vi "PSUSettingsMenu.vi"(8 "error in (no error)":errorcluster, 9 "PSU Calc":T1={"Low speed (km/s)"=2000.0, "High speed (km/s)"=3000.0, "Window (Delta-T)"=0.0, "Lower Cutoff"=0.0, "Multiplier"=0, "Low Charge (fC)"=2000.0, "High Charge (fC)"=2000.0, "High Mass (kg)"=2000.0, "Low Mass (kg)"=2000.0, "High Radius (µm) "=0.0, "Low Radius (µm)"=2000.0, "Exp. Voltage (MV)"=2000.0} {"Exp. Voltage (MV)" step=0.01 format="%#.6f"; "Window (Delta-T)" step=1.0 format="%#.0f"; "High Radius (µm)" min=0.0 max=1000.0; "High Mass (kg)" min=0.0 max=1.0; "High Charge (fC)" min=0.0 max=1000000000000.0; "High speed (km/s)" min=0.0 max=299790.0; "Low speed (km/s)" min=0.0 max=299790.0; "Low Charge (fC)" min=0.0 max=1000000000000.0; "Low Mass (kg)" min=0.0 max=1.0; "Low Radius (µm)" min=0.0 max=299792000.0; "Lower Cutoff" step=1.0 format="%#.0f"; "Multiplier" items=["1k", "10k"]}, 10 "sub vi?":bool, 11 "Enable":bool=TRUE) -> (0 "error out":errorcluster, 1 "OK":bool, 3 "Cancel 2":bool caption="Cancel")   [LabVIEW 2013]
doc: "Displays a standard dialog box that prompts users to enter information, such as a user name and password.\n--------------------\n\nThis Express VI is configured as follows:\n\nMessage to Display to the User:Please Enter Experiment Settings Information For Database Storage.\nThe inputs are: \nNumber: Please Enter Group ID\nText Entry Box: Please Enter Tags:\nText Entry Box: Please Enter Experiment Description:"
uses:
  Controls/PSU Calc.ctl
  <vilib>/Utility/miscctls.llb/LVPointTypeDef.ctl
  <vilib>/addons/database/Connection.llb/Conn Execute.vi
  <vilib>/addons/database/Recordset.llb/Rec Fetch Recordset Data (R).vi
  <vilib>/addons/database/Recordset.llb/Rec Destroy - Connection.vi
  Unused/PSU updated.vi
  <vilib>/addons/database/_DB Variant To Data/Database Variant To Data.xnode
  <vilib>/addons/database/NI_Database_API.lvlib
panel:
  in  "Accept All Particles":bool caption="OK2"
  out "Dust Density\n(g/cc)":dbl
  in  "Variable 2":enum32{"Velocity", "Charge", "Mass"}(radio)
  in  "Variable 1":enum32{"Velocity", "Charge", "Mass"}(radio)
  in  "PSU update":bool caption="OK2"
  in  "Cancel":bool
  in  "OK1":bool
  # "Please Enter PSU Settings For Storage in the CCLDAS Database."
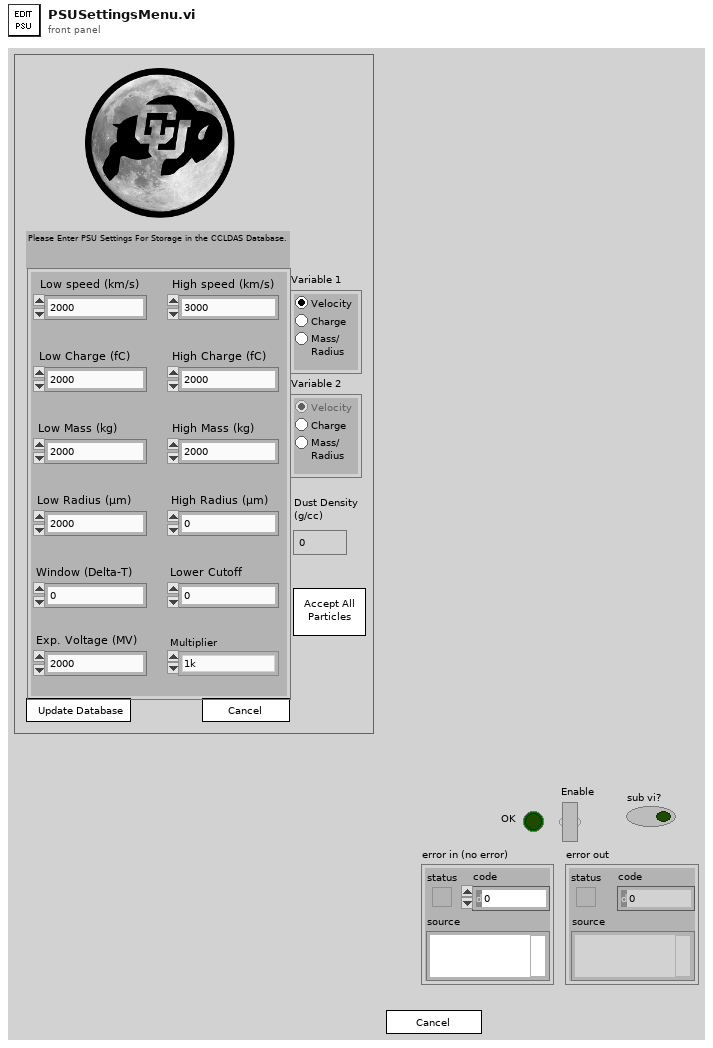
[diagram p1: front panel]
types:
  T1 = typedef "PSU Calc.ctl" = cluster{"Low speed (km/s)":dbl, "High speed (km/s)":dbl, "Window (Delta-T)":dbl, "Lower Cutoff":dbl, "Multiplier":u16, "Low Charge (fC)":dbl, "High Charge (fC)":dbl, "High Mass (kg)":dbl, "Low Mass (kg)":dbl, "High Radius (µm) ":dbl, "Low Radius (µm)":dbl, "Exp. Voltage (MV)":dbl}
  T2 = typedef "LVPointTypeDef.ctl" = cluster{"Horizontal":i16, "Vertical":i16}
  T3 = enum32{"Invalid", "Standard", "Closed", "Hidden", "Minimized", "Maximized"}
  T4 = enum8{"Enabled", "Disabled", "Disabled and Grayed Out"}
  T5 = cluster{"Integer Timestamp":dbl, "Max Velocity":dbl, "Min Velocity":dbl, "Max Charge":dbl, "Min Charge":dbl, "Max Mass":dbl, "Min Mass":dbl, "Variable 1":enum8{"Velocity", "Charge", "Mass"}, "Variable 2":enum8{"Velocity", "Charge", "Mass"}}
  T6 = typedef "NI_Database_API.lvlib/Conn ObjectReference.ctl" = refnum<k1>
  T7 = typedef "NI_Database_API.lvlib/Rec ObjectReference.ctl" = refnum<k1>
  T8 = cluster{"Integer Timestamp":dbl, "Max Velocity":dbl, "Min Velocity":dbl, "Max Charge":dbl, "Min Charge":dbl, "Max Mass":dbl, "Min Mass":dbl, "Variable 1":enum32{"Velocity", "Charge", "Mass", "Radius"}, "Variable 2":enum32{"Velocity", "Charge", "Mass", "Radius"}}
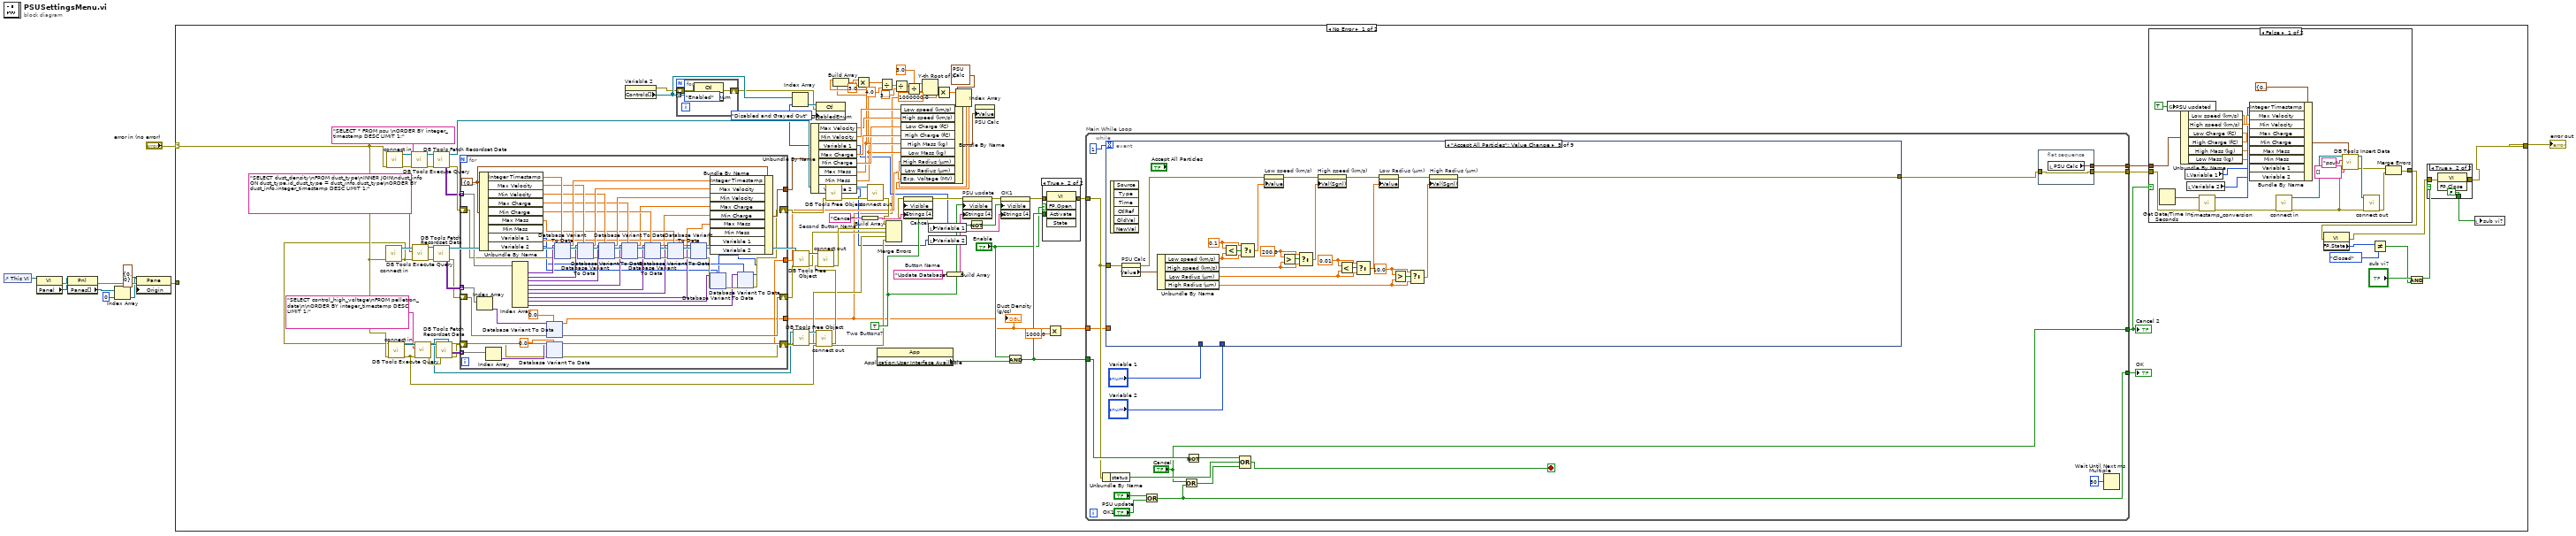
[diagram p0: block diagram]
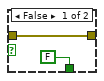
[diagram p2: hidden frame]
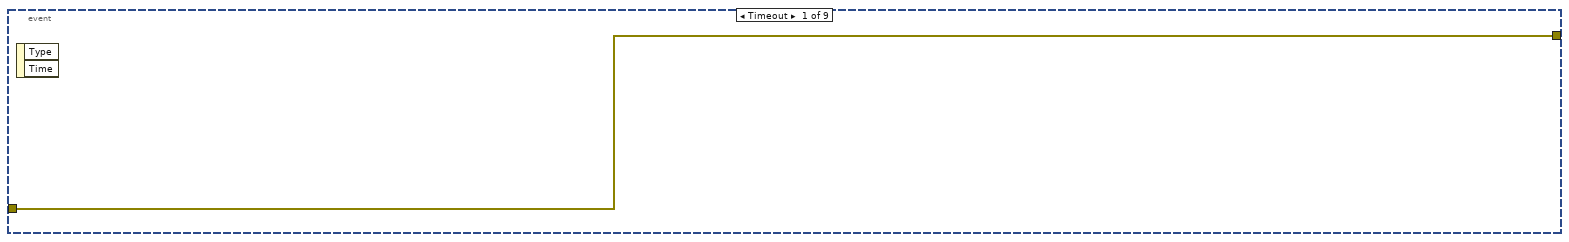
[diagram p5: hidden frame]
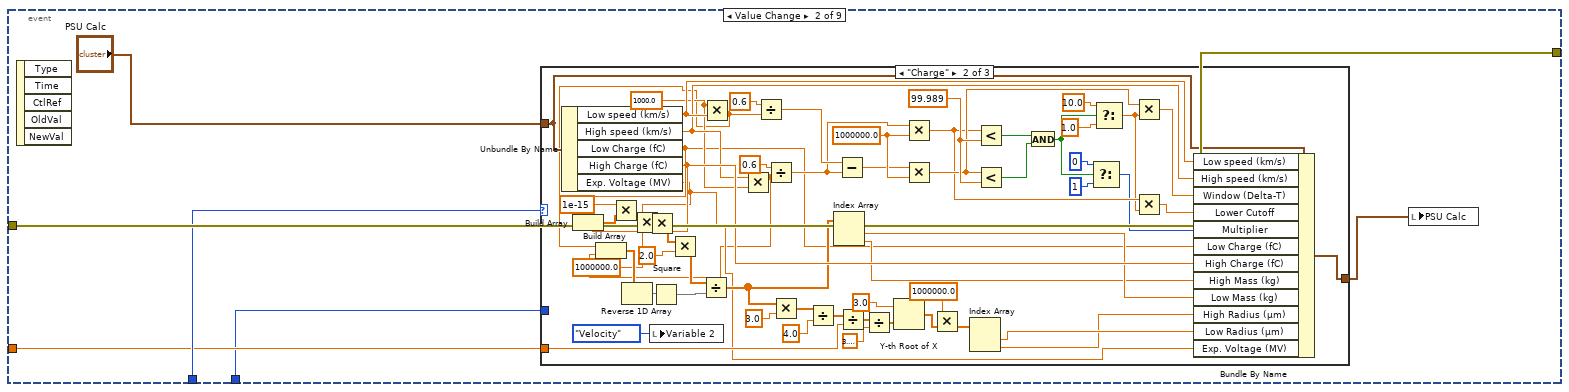
[diagram p6: hidden frame]
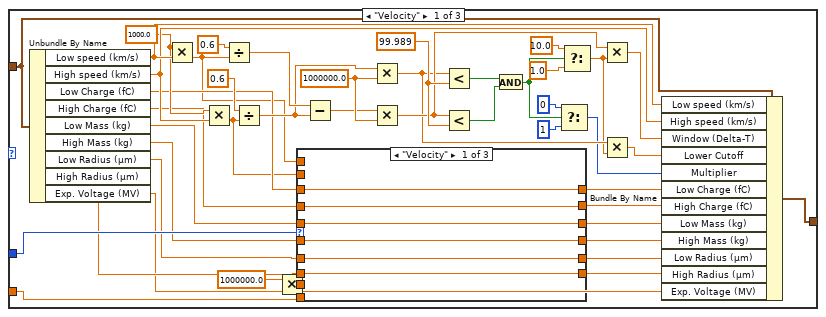
[diagram p7: hidden frame]
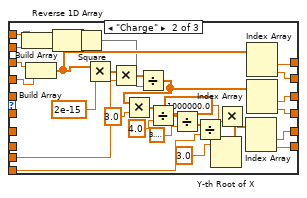
[diagram p8: hidden frame]
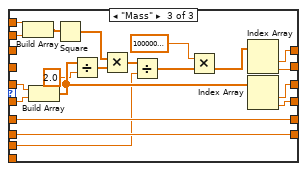
[diagram p9: hidden frame]
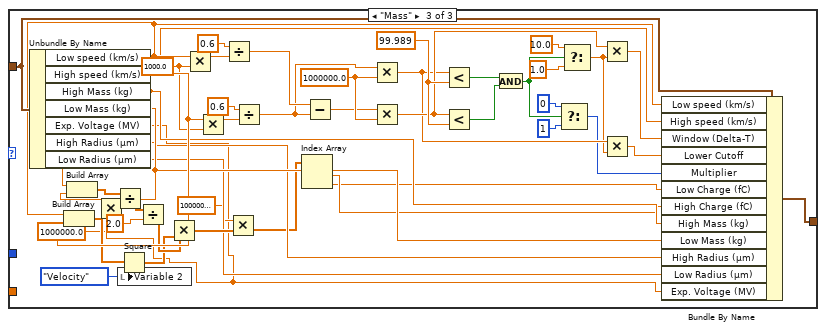
[diagram p10: hidden frame]
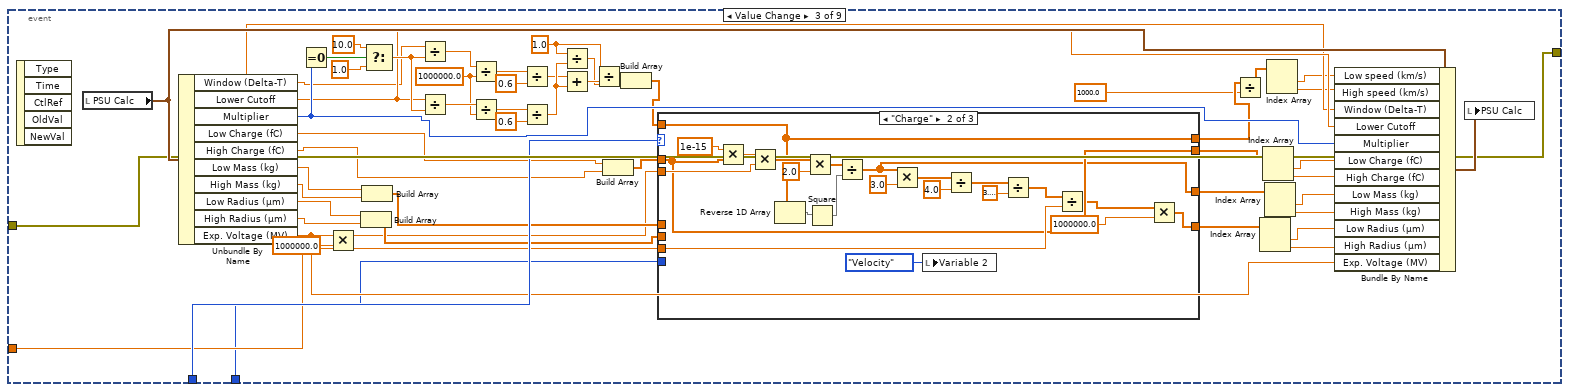
[diagram p11: hidden frame]
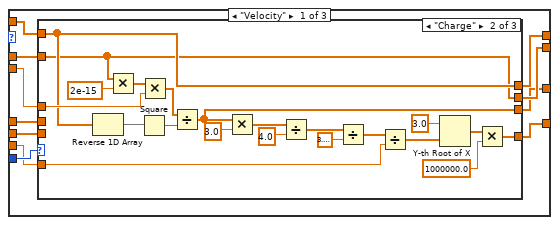
[diagram p12: hidden frame]
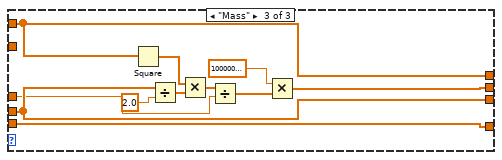
[diagram p14: hidden frame]
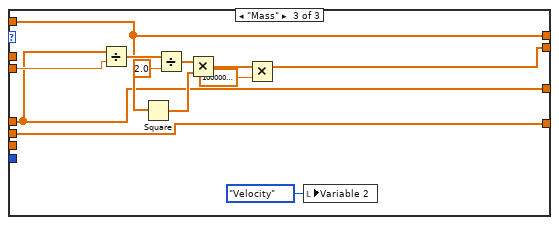
[diagram p15: hidden frame]
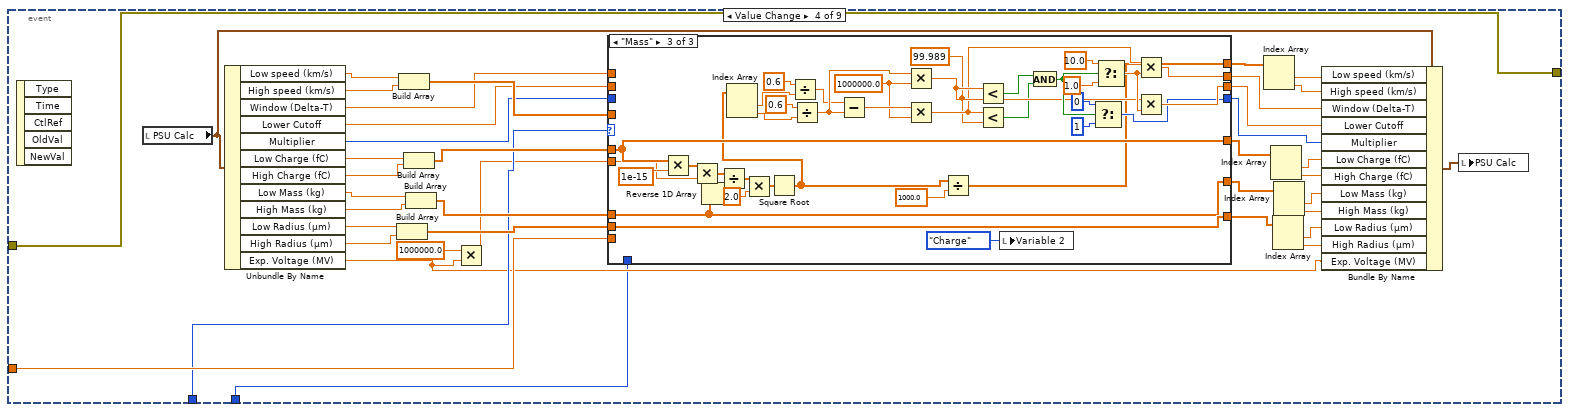
[diagram p16: hidden frame]
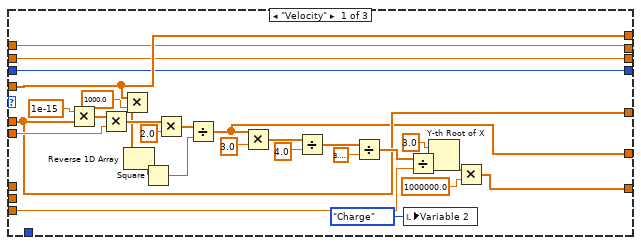
[diagram p17: hidden frame]
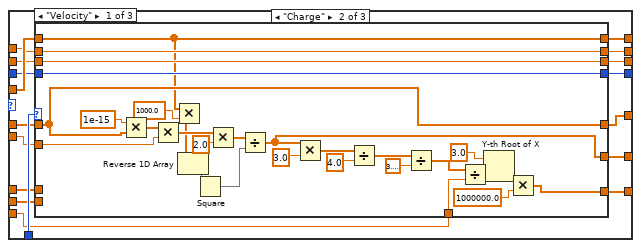
[diagram p18: hidden frame]
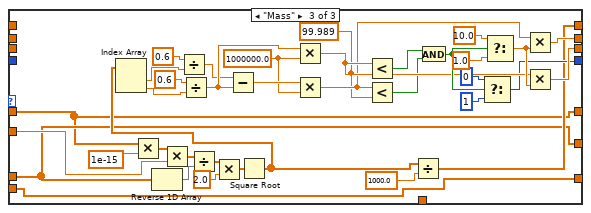
[diagram p20: hidden frame]
diagram:
  n1 = control-ref of="This VI"() -> (w9:refnum<vi>)
  n2 = property class="VI"(reference=w9) -> (error out=w8:errorcluster, "Panel"=w7:refnum<vi>)  [unwired: 1 in, 1 out]
  n3 = property class="Pnl"(reference=w7, error in=w8) -> (error out=w6:errorcluster, "Panes[]"=w5:refnum<vi>[])  [unwired: 1 out]
  n4 = Index Array(array=w5, index=0) -> (element=w3:refnum<vi>)
  n5 = property class="Pane"(reference=w3, error in=w6, "Origin"=T2 {"Horizontal"=0, "Vertical"=0}) -> (error out=w1:errorcluster)  [unwired: 1 out]
  n6 = case shown="No Error" "error in (no error)" {
    selector: "error in (no error)" -> [w72 w1751]
    tunnel: [w23 w1751] -> w10
    tunnel: w1 -> [_ _]
    frame No Error {
      w94 = "Cancel"  # Second Button Name
      w96 = "Update Database"  # Button Name
      w88 = TRUE  # Two Buttons?
      n7 = call "connect in.vi"("error in (no error)"=w72) -> ("error out"=w58:errorcluster, "Database Connection"=w78:T6)  [unwired: 6 in, 1 out]
      n8 = call "connect in.vi"("error in (no error)"=w72) -> ("error out"=w101:errorcluster, "Database Connection"=w100:T6)  [unwired: 6 in, 1 out]
      n9 = call "connect in.vi"("error in (no error)"=w72) -> ("error out"=w59:errorcluster, "Database Connection"=w71:T6)  [unwired: 6 in, 1 out]
      n10 = call-poly <vilib>:"DB Tools Execute Query.vi"("error in (no error)"=w101, "SQL query"="SELECT * FROM psu \nORDER BY integer_timestamp DESC LIMIT 1;", "connection reference"=w100) -> ("error out"=w103:errorcluster, "recordset reference"=w102:T7)  [unwired: 5 in]
      n11 = call-poly <vilib>:"DB Tools Execute Query.vi"("error in (no error)"=w58, "SQL query"="SELECT dust_density\nFROM dust_type\nINNER JOIN\ndust_info ON dust_type.id_dust_type = dust_info.dust_type\nORDER BY dust_info.integer_timestamp DESC LIMIT 1;", "connection reference"=w78) -> ("error out"=w75:errorcluster, "recordset reference"=w76:T7)  [unwired: 5 in]
      n12 = call-poly <vilib>:"DB Tools Execute Query.vi"("error in (no error)"=w59, "SQL query"="SELECT control_high_voltage\nFROM pelletron_data\n\nORDER BY integer_timestamp DESC LIMIT 1;", "connection reference"=w71) -> ("error out"=w70:errorcluster, "recordset reference"=w69:T7)  [unwired: 5 in]
      n13 = call-poly <vilib>:"DB Tools Fetch Recordset Data.vi"("error in (no error)"=w103, "recordset reference"=w102) -> ("error out"=w109:errorcluster, "recordset data"=w108:variant[][], "recordset reference out"=w104:T7)  [unwired: 3 in]
      n14 = call-poly <vilib>:"DB Tools Fetch Recordset Data.vi"("error in (no error)"=w75, "recordset reference"=w76) -> ("error out"=w73:errorcluster, "recordset data"=w74:variant[][], "recordset reference out"=w62:T7)  [unwired: 3 in]
      n15 = call-poly <vilib>:"DB Tools Fetch Recordset Data.vi"("error in (no error)"=w70, "recordset reference"=w69) -> ("error out"=w66:errorcluster, "recordset data"=w68:variant[][], "recordset reference out"=w63:T7)  [unwired: 3 in]
      n16 = for {
        tunnel: w108 -> [w199] mode=indexing
        shift-right: [w158] -> w82
        shift-left: w109 -> [w195]
        tunnel: [w194] -> w87
        tunnel: w74 -> [w168] mode=indexing
        shift-right: [w162] -> w65
        shift-left: w73 -> [w163]
        tunnel: w68 -> [w167] mode=indexing
        shift-right: [w161] -> w64
        shift-left: w66 -> [w164]
        tunnel: [w150] -> w47
        tunnel: [w148] -> w14
        w189 = T8 {"Integer Timestamp"=0.0, "Max Velocity"=0.0, "Min Velocity"=0.0, "Max Charge"=0.0, "Min Charge"=0.0, "Max Mass"=0.0, "Min Mass"=0.0, "Variable 1"=enum."Velocity", "Variable 2"=enum."Velocity"} ("PSU settings")
        n17 = Index Array(array=w168) -> (element=w166:variant)  [unwired: 1 in]
        n18 = Unbundle By Name(w189) -> ("Integer Timestamp"=w193:dbl, "Max Velocity"=w190:dbl, "Min Velocity"=w187:dbl, "Max Charge"=w176:dbl, "Min Charge"=w175:dbl, "Max Mass"=w174:dbl, "Min Mass"=w173:dbl, "Variable 1"=w155:enum32{"Velocity", "Charge", "Mass", "Radius"}, "Variable 2"=w154:enum32{"Velocity", "Charge", "Mass", "Radius"})
        n19 = Index Array(array=w167) -> (element=w165:variant)  [unwired: 1 in]
        n20 = Index Array(array=w199) -> (element #1=w198:variant, element #2=w197:variant, element #3=w188:variant, element #4=w181:variant, element #5=w180:variant, element #6=w179:variant, element #7=w177:variant, element #8=w157:variant, element #9=w156:variant)  [unwired: 9 in]
        n21 = xnode "Database Variant To Data"("database variant"=w166, "error in (no error)"=w163, "type"=0.0) -> ("data"=w148:dbl, "error out"=w162:errorcluster)
        n22 = xnode "Database Variant To Data"("database variant"=w165, "error in (no error)"=w164, "type"=0.0) -> ("data"=w150:dbl, "error out"=w161:errorcluster)
        n23 = xnode "Database Variant To Data"("database variant"=w198, "error in"=w195, "type"=w193) -> ("data"=w192:dbl, "error out"=w196:errorcluster)
        n24 = xnode "Database Variant To Data"("database variant"=w197, "error in"=w196, "type"=w190) -> ("data"=w191:dbl, "error out"=w185:errorcluster)
        n25 = xnode "Database Variant To Data"("database variant"=w188, "error in"=w185, "type"=w187) -> ("data"=w186:dbl, "error out"=w182:errorcluster)
        n26 = xnode "Database Variant To Data"("database variant"=w181, "error in (no error)"=w182, "type"=w176) -> ("data"=w172:dbl, "error out"=w184:errorcluster)
        n27 = xnode "Database Variant To Data"("database variant"=w180, "error in (no error)"=w184, "type"=w175) -> ("data"=w171:dbl, "error out"=w183:errorcluster)
        n28 = xnode "Database Variant To Data"("database variant"=w179, "error in (no error)"=w183, "type"=w174) -> ("data"=w170:dbl, "error out"=w178:errorcluster)
        n29 = xnode "Database Variant To Data"("database variant"=w177, "error in (no error)"=w178, "type"=w173) -> ("data"=w169:dbl, "error out"=w159:errorcluster)
        n30 = xnode "Database Variant To Data"("database variant"=w157, "error in (no error)"=w159, "type"=w155) -> ("data"=w153:enum32{"Velocity", "Charge", "Mass", "Radius"}, "error out"=w160:errorcluster)
        n31 = xnode "Database Variant To Data"("database variant"=w156, "error in (no error)"=w160, "type"=w154) -> ("data"=w152:enum32{"Velocity", "Charge", "Mass", "Radius"}, "error out"=w158:errorcluster)
        n32 = Bundle By Name(cluster=w189, "Integer Timestamp"=w192, "Max Velocity"=w191, "Min Velocity"=w186, "Max Charge"=w172, "Min Charge"=w171, "Max Mass"=w170, "Min Mass"=w169, "Variable 1"=w153, "Variable 2"=w152) -> (w194:T8)
      }
      "Dust Density\n(g/cc)" <- w14
      n33 = property on="Variable 2" class="RadioBtnsControl (strict)"() -> (error out=w29:errorcluster, "Controls[]"=w30:refnum<vi>[])  [unwired: 2 in, 1 out]
      n34 = for {
        tunnel: w30 -> [w122] mode=indexing
        shift-right: [w119] -> w28
        shift-left: w29 -> [w121]
        n35 = property class="Ctl"(reference=w122, error in=w121, "DisabledEnum"=T4."Enabled" ("Disabled")) -> (error out=w119:errorcluster)  [unwired: 1 out]
      }
      n36 = call-poly <vilib>:"DB Tools Free Object.vi"("error in (no error)"=w65, "recordset reference"=w62) -> ("error out"=w56:errorcluster, "connection reference"=w61:T6)  [unwired: 8 in]
      n37 = call-poly <vilib>:"DB Tools Free Object.vi"("error in (no error)"=w64, "recordset reference"=w63) -> ("error out"=w54:errorcluster, "connection reference"=w60:T6)  [unwired: 8 in]
      n38 = Unbundle By Name(w87) -> ("Max Velocity"=w83:dbl, "Min Velocity"=w84:dbl, "Variable 1"=w27:enum32{"Velocity", "Charge", "Mass", "Radius"}, "Max Charge"=w49:dbl, "Min Charge"=w48:dbl, "Max Mass"=w46:dbl, "Min Mass"=w45:dbl, "Variable 2"=w26:enum32{"Velocity", "Charge", "Mass", "Radius"})
      n39 = Index Array(array=w30, index=w27) -> (element=w51:refnum<vi>)
      n40 = property class="Ctl"(reference=w51, error in=w28, "DisabledEnum"=T4."Disabled and Grayed Out" ("Disabled")) -> ()  [unwired: 2 out]
      n41 = call "connect out.vi"("error in (no error)"=w59, "connection reference"=w60) -> ("error out"=w55:errorcluster)  [unwired: 9 in]
      n42 = call "connect out.vi"("error in (no error)"=w58, "connection reference"=w61) -> ("error out"=w57:errorcluster)  [unwired: 9 in]
      n43 = call-poly <vilib>:"DB Tools Free Object.vi"("error in (no error)"=w82, "recordset reference"=w104) -> ("error out"=w105:errorcluster, "connection reference"=w106:T6)  [unwired: 8 in]
      n44 = Build Array(w46, w45) -> (w44:dbl[])
      n45 = Multiply(x=w44, y=3.0 ("Min Mass")) -> (x*y=w42:dbl[])
      n46 = Build Array(w94) -> (w93:string[])
      n47 = call "connect out.vi"("error in (no error)"=w105, "connection reference"=w106) -> ("error out"=w53:errorcluster)  [unwired: 9 in]
      n48 = property class="App"() -> ("Application:User Interface Available"=w98:bool)  [unwired: 2 in, 2 out]
      n49 = Divide(x=w42, y=4.0 ("Min Mass")) -> (x/y=w40:dbl[])
      n50 = Merge Errors(w53, w57, w56, w54, w55) -> (w52:errorcluster)
      n51 = Divide(x=w40, y=3.141592653589793) -> (x/y=w38:dbl[])
      n52 = property on="Cancel" class="Bool"(error in=w52, "Visible"=w88, "Strings [4]"=w93) -> (error out=w91:errorcluster)  [unwired: 1 in, 1 out]
      n53 = Divide(x=w38, y=w14) -> (x/y=w37:dbl[])
      n54 = Y-th Root of X(1:w37, 2:3.0 ("Min Mass")) -> (0:w33:dbl[])
      n55 = local write "Variable 1"(w27) -> ()
      n56 = local write "Variable 2"(w26) -> ()
      n57 = Multiply(x=w33, y=1000000.0 ("Min Mass")) -> (x*y=w32:dbl[])
      n58 = Build Array(w96) -> (w95:string[])
      n59 = Index Array(array=w32) -> (element #1=w36:dbl, element #2=w35:dbl)  [unwired: 2 in]
      n60 = Bundle By Name(cluster=T1 {"Low speed (km/s)"=2000.0, "High speed (km/s)"=3000.0, "Window (Delta-T)"=0.0, "Lower Cutoff"=0.0, "Multiplier"=0, "Low Charge (fC)"=0.0, "High Charge (fC)"=0.0, "High Mass (kg)"=0.0, "Low Mass (kg)"=0.0, "High Radius (µm) "=0.0, "Low Radius (µm)"=0.0, "Exp. Voltage (MV)"=0.0} ("PSU Calc"), "Low speed (km/s)"=w84, "High speed (km/s)"=w83, "Low Charge (fC)"=w48, "High Charge (fC)"=w49, "High Mass (kg)"=w46, "Low Mass (kg)"=w45, "High Radius (µm)"=w36, "Low Radius (µm)"=w35, "Exp. Voltage (MV)"=w47) -> (w86:T1)
      n61 = property on="PSU update" class="Bool"(error in=w91, "Visible"=w88, "Strings [4]"=w95) -> (error out=w92:errorcluster)  [unwired: 1 in, 1 out]
      n62 = Not(x=w88) -> (.not. x?=w90:bool)
      n63 = property on="PSU Calc" class="Clust (strict)"("Value"=w86) -> ()  [unwired: 2 in, 2 out]
      n64 = property on="OK1" class="Bool"(error in=w92, "Visible"=w90, "Strings [4]"=w95) -> (error out=w97:errorcluster)  [unwired: 1 in, 1 out]
      n65 = And(x="Enable", y=w98) -> (x .and. y?=w25:bool)
      n66 = case shown="True" "Enable" {
        tunnel: [w115 w118] -> w99
        tunnel: w97 -> [w115 w117]
        tunnel: w25 -> [_ w116]
        frame False {
        }
        frame True {
          n67 = invoke class="VI" method="FP.Open"(error in=w117, "Activate"=w116) -> (error out=w118:errorcluster)  [unwired: 3 in, 4 out]
        }
      }
      n68 = Multiply(x=w14, y=1000.0) -> (x*y=w13:dbl)
      n69 = while "Main While Loop" {
        tunnel: [w567] -> w89
        tunnel: w25 -> [w565]
        tunnel: w99 -> [w559]
        tunnel: [w557] -> w80
        tunnel: ["Cancel"] -> w81
        tunnel: [w555] -> w79
        tunnel: w13 -> [w553]
        stop <- w561 stop-if-true
        n70 = Unbundle By Name(w559) -> ("status"=w562:bool)
        n71 = event shown="[8] \"Accept All Particles\": Value Change" {
          selector: _ -> [_ _ _ _ _ _ _ _ _]
          dyn-events: _ -> [_ _ _ _ _ _ _ _ _]
          timeout: 1 -> [_ _ _ _ _ _ _ _ _]
          tunnel: w559 -> [w572 w577 w835 w923 w1115 w1387 w1398 w1566 w1750]
          tunnel: [w572 w577 w835 w923 w1115 w1379 w1398 w1566 w1728] -> w556
          tunnel: "Variable 1" -> [_ w575 w816 w924 w1116 _ w1412 w1582 _]
          tunnel: w553 -> [_ w574 w809 w943 w1136 _ w1404 w1575 _]
          tunnel: "Variable 2" -> [_ w573 w785 w919 w1117 w1383 w1394 w1562 _]
          event Timeout {
            n72 = event-data() -> ()  [unwired: 1 in, 2 out]
          }
          event Value Change {
            n73 = event-data() -> ()  [unwired: 1 in, 5 out]
            n74 = case shown="\"Charge\"" w575 {
              tunnel: [w622 w738 w784] -> w578
              tunnel: "PSU Calc" -> [w621 w737 w783]
              tunnel: w574 -> [w581 w699 _]
              tunnel: w573 -> [w597 _ _]
              frame "Velocity" {
                w598 = 1000.0 ("x")
                w612 = 99.989
                w614 = 1000000.0 ("y")
                n75 = Unbundle By Name(w621) -> ("Low speed (km/s)"=w603:dbl, "High speed (km/s)"=w599:dbl, "Low Charge (fC)"=w596:dbl, "High Charge (fC)"=w594:dbl, "Low Mass (kg)"=w592:dbl, "High Mass (kg)"=w591:dbl, "Low Radius (µm)"=w588:dbl, "High Radius (µm)"=w586:dbl, "Exp. Voltage (MV)"=w584:dbl)
                n76 = Multiply(x=w598, y=w603) -> (x*y=w582:dbl)
                n77 = Multiply(x=w598, y=w599) -> (x*y=w583:dbl)
                n78 = Divide(x=0.6, y=w582) -> (x/y=w616:dbl)
                n79 = Divide(x=0.6, y=w583) -> (x/y=w615:dbl)
                n80 = Multiply(x=1000000.0, y=w584) -> (x*y=w580:dbl)
                n81 = case shown="\"Velocity\"" w597 {
                  tunnel: w596 -> [w628 w656 _]
                  tunnel: [w628 w655 w673] -> w595
                  tunnel: w594 -> [w627 w657 _]
                  tunnel: [w627 w650 w670] -> w593
                  tunnel: w592 -> [w626 _ w677]
                  tunnel: [w626 w654 w672] -> w590
                  tunnel: w591 -> [w625 _ w676]
                  tunnel: [w625 w653 w671] -> w589
                  tunnel: w588 -> [w624 _ w675]
                  tunnel: [w624 w652 w675] -> w587
                  tunnel: w586 -> [w623 _ w674]
                  tunnel: [w623 w651 w674] -> w585
                  tunnel: w580 -> [_ w646 w663]
                  tunnel: w583 -> [_ w658 w678]
                  tunnel: w582 -> [_ w659 w679]
                  tunnel: w581 -> [_ w633 _]
                  frame "Velocity" {
                  }
                  frame "Charge" {
                    n82 = Build Array(w659, w658) -> (w644:dbl[])
                    n83 = Build Array(w656, w657) -> (w649:dbl[])
                    n84 = Reverse 1D Array(array=w644) -> (reversed array=w629:dbl[])
                    n85 = Square(x=w629) -> (x^2=w643:dbl[])
                    n86 = Multiply(x=w649, y=2e-15 ("x")) -> (x*y=w647:dbl[])
                    n87 = Multiply(x=w647, y=w646) -> (x*y=w645:dbl[])
                    n88 = Divide(x=w645, y=w643) -> (x/y=w642:dbl[])
                    n89 = Multiply(x=w642, y=3.0 ("x")) -> (x*y=w640:dbl[])
                    n90 = Divide(x=w640, y=4.0 ("x")) -> (x/y=w639:dbl[])
                    n91 = Divide(x=w639, y=3.141592653589793) -> (x/y=w638:dbl[])
                    n92 = Divide(x=w638, y=w633) -> (x/y=w637:dbl[])
                    n93 = Y-th Root of X(1:w637, 2:3.0 ("x")) -> (0:w632:dbl[])
                    n94 = Multiply(x=w632, y=1000000.0 ("x")) -> (x*y=w631:dbl[])
                    n95 = Index Array(array=w631) -> (element #1=w652:dbl, element #2=w651:dbl)  [unwired: 2 in]
                    n96 = Index Array(array=w649) -> (element #1=w655:dbl, element #2=w650:dbl)  [unwired: 2 in]
                    n97 = Index Array(array=w642) -> (element #1=w654:dbl, element #2=w653:dbl)  [unwired: 2 in]
                  }
                  frame "Mass" {
                    n98 = Build Array(w679, w678) -> (w669:dbl[])
                    n99 = Build Array(w677, w676) -> (w668:dbl[])
                    n100 = Square(x=w669) -> (x^2=w665:dbl[])
                    n101 = Divide(x=w668, y=2.0 ("x")) -> (x/y=w666:dbl[])
                    n102 = Multiply(x=w665, y=w666) -> (x*y=w664:dbl[])
                    n103 = Divide(x=w664, y=w663) -> (x/y=w662:dbl[])
                    n104 = Multiply(x=1000000000000000.0, y=w662) -> (x*y=w661:dbl[])
                    n105 = Index Array(array=w661) -> (element #1=w673:dbl, element #2=w670:dbl)  [unwired: 2 in]
                    n106 = Index Array(array=w668) -> (element #1=w672:dbl, element #2=w671:dbl)  [unwired: 2 in]
                  }
                }
                n107 = Subtract(x=w616, y=w615) -> (x-y=w613:dbl)
                n108 = Multiply(x=w615, y=w614) -> (x*y=w606:dbl)
                n109 = Multiply(x=w613, y=w614) -> (x*y=w607:dbl)
                n110 = Less?(x=w606, y=w612) -> (x < y?=w611:bool)
                n111 = Less?(x=w607, y=w612) -> (x < y?=w610:bool)
                n112 = And(x=w611, y=w610) -> (x .and. y?=w604:bool)
                n113 = Select(t=u16 0 ("Multiplier"), s=w604, f=u16 1 ("Multiplier")) -> (s? t:f=w600:u16)
                n114 = Select(t=10.0, s=w604, f=1.0) -> (s? t:f=w605:dbl)
                n115 = Multiply(x=w607, y=w605) -> (x*y=w619:dbl)
                n116 = Multiply(x=w606, y=w605) -> (x*y=w620:dbl)
                n117 = Bundle By Name(cluster=w621, "Low speed (km/s)"=w603, "High speed (km/s)"=w599, "Window (Delta-T)"=w619, "Lower Cutoff"=w620, "Multiplier"=w600, "Low Charge (fC)"=w595, "High Charge (fC)"=w593, "Low Mass (kg)"=w590, "High Mass (kg)"=w589, "Low Radius (µm)"=w587, "High Radius (µm)"=w585, "Exp. Voltage (MV)"=w584) -> (w622:T1)
              }
              frame "Charge" {
                w687 = 1000.0 ("x")
                w728 = 99.989
                w730 = 1000000.0 ("y")
                n118 = Unbundle By Name(w737) -> ("Low speed (km/s)"=w711:dbl, "High speed (km/s)"=w710:dbl, "Low Charge (fC)"=w686:dbl, "High Charge (fC)"=w715:dbl, "Exp. Voltage (MV)"=w685:dbl)
                n119 = Build Array(w686, w715) -> (w714:dbl[])
                n120 = Multiply(x=1e-15, y=w714) -> (x*y=w691:dbl[])
                n121 = Multiply(x=w685, y=1000000.0) -> (x*y=w684:dbl)
                n122 = Multiply(x=w691, y=w684) -> (x*y=w713:dbl[])
                n123 = local write "Variable 2"(enum32{"Velocity", "Charge", "Mass"}."Velocity" ("Variable 2")) -> ()
                n124 = Multiply(x=w713, y=2.0) -> (x*y=w708:dbl[])
                n125 = Multiply(x=w687, y=w711) -> (x*y=w682:dbl)
                n126 = Multiply(x=w710, y=w687) -> (x*y=w681:dbl)
                n127 = Build Array(w682, w681) -> (w709:dbl[])
                n128 = Reverse 1D Array(array=w709) -> (reversed array=w680:dbl[])
                n129 = Square(x=w680) -> (x^2=w707:dbl[])
                n130 = Divide(x=w708, y=w707) -> (x/y=w704:dbl[])
                n131 = Divide(x=0.6, y=w682) -> (x/y=w732:dbl)
                n132 = Divide(x=0.6, y=w681) -> (x/y=w731:dbl)
                n133 = Multiply(x=w704, y=3.0) -> (x*y=w702:dbl[])
                n134 = Divide(x=w702, y=4.0) -> (x/y=w700:dbl[])
                n135 = Index Array(array=w704) -> (element #1=w706:dbl, element #2=w705:dbl)  [unwired: 2 in]
                n136 = Subtract(x=w732, y=w731) -> (x-y=w729:dbl)
                n137 = Divide(x=w700, y=w699) -> (x/y=w698:dbl[])
                n138 = Divide(x=w698, y=3.141592653589793) -> (x/y=w696:dbl[])
                n139 = Y-th Root of X(1:w696, 2:3.0) -> (0:w694:dbl[])
                n140 = Multiply(x=w731, y=w730) -> (x*y=w722:dbl)
                n141 = Multiply(x=w729, y=w730) -> (x*y=w723:dbl)
                n142 = Multiply(x=1000000.0, y=w694) -> (x*y=w689:dbl[])
                n143 = Index Array(array=w689) -> (element #1=w693:dbl, element #2=w692:dbl)  [unwired: 2 in]
                n144 = Less?(x=w722, y=w728) -> (x < y?=w727:bool)
                n145 = Less?(x=w723, y=w728) -> (x < y?=w726:bool)
                n146 = And(x=w727, y=w726) -> (x .and. y?=w720:bool)
                n147 = Select(t=u16 0 ("Multiplier"), s=w720, f=u16 1 ("Multiplier")) -> (s? t:f=w717:u16)
                n148 = Select(t=10.0, s=w720, f=1.0) -> (s? t:f=w721:dbl)
                n149 = Multiply(x=w723, y=w721) -> (x*y=w735:dbl)
                n150 = Multiply(x=w722, y=w721) -> (x*y=w736:dbl)
                n151 = Bundle By Name(cluster=w737, "Low speed (km/s)"=w711, "High speed (km/s)"=w710, "Window (Delta-T)"=w735, "Lower Cutoff"=w736, "Multiplier"=w717, "Low Charge (fC)"=w686, "High Charge (fC)"=w715, "High Mass (kg)"=w705, "Low Mass (kg)"=w706, "High Radius (µm)"=w692, "Low Radius (µm)"=w693, "Exp. Voltage (MV)"=w685) -> (w738:T1)
              }
              frame "Mass" {
                w742 = 1000.0 ("y")
                w774 = 99.989
                w776 = 1000000.0 ("y")
                n152 = Unbundle By Name(w783) -> ("Low speed (km/s)"=w759:dbl, "High speed (km/s)"=w758:dbl, "High Mass (kg)"=w753:dbl, "Low Mass (kg)"=w752:dbl, "Exp. Voltage (MV)"=w741:dbl, "High Radius (µm)"=w748:dbl, "Low Radius (µm)"=w747:dbl)
                n153 = Build Array(w759, w758) -> (w757:dbl[])
                n154 = Build Array(w753, w752) -> (w749:dbl[])
                n155 = Multiply(x=w741, y=1000000.0) -> (x*y=w740:dbl)
                n156 = Divide(x=w749, y=w740) -> (x/y=w761:dbl[])
                n157 = local write "Variable 2"(enum32{"Velocity", "Charge", "Mass"}."Velocity" ("Variable 2")) -> ()
                n158 = Square(x=w757) -> (x^2=w755:dbl[])
                n159 = Divide(x=w761, y=2.0) -> (x/y=w756:dbl[])
                n160 = Multiply(x=w756, y=w755) -> (x*y=w754:dbl[])
                n161 = Multiply(x=w759, y=w742) -> (x*y=w744:dbl)
                n162 = Multiply(x=w758, y=w742) -> (x*y=w743:dbl)
                n163 = Divide(x=0.6, y=w744) -> (x/y=w778:dbl)
                n164 = Multiply(x=1000000000000000.0, y=w754) -> (x*y=w746:dbl[])
                n165 = Divide(x=0.6, y=w743) -> (x/y=w777:dbl)
                n166 = Index Array(array=w746) -> (element #1=w751:dbl, element #2=w750:dbl)  [unwired: 2 in]
                n167 = Subtract(x=w778, y=w777) -> (x-y=w775:dbl)
                n168 = Multiply(x=w777, y=w776) -> (x*y=w768:dbl)
                n169 = Multiply(x=w775, y=w776) -> (x*y=w769:dbl)
                n170 = Less?(x=w768, y=w774) -> (x < y?=w773:bool)
                n171 = Less?(x=w769, y=w774) -> (x < y?=w772:bool)
                n172 = And(x=w773, y=w772) -> (x .and. y?=w766:bool)
                n173 = Select(t=u16 0 ("Multiplier"), s=w766, f=u16 1 ("Multiplier")) -> (s? t:f=w763:u16)
                n174 = Select(t=10.0, s=w766, f=1.0) -> (s? t:f=w767:dbl)
                n175 = Multiply(x=w769, y=w767) -> (x*y=w781:dbl)
                n176 = Multiply(x=w768, y=w767) -> (x*y=w782:dbl)
                n177 = Bundle By Name(cluster=w783, "Low speed (km/s)"=w759, "High speed (km/s)"=w758, "Window (Delta-T)"=w781, "Lower Cutoff"=w782, "Multiplier"=w763, "Low Charge (fC)"=w750, "High Charge (fC)"=w751, "High Mass (kg)"=w753, "Low Mass (kg)"=w752, "High Radius (µm)"=w748, "Low Radius (µm)"=w747, "Exp. Voltage (MV)"=w741) -> (w784:T1)
              }
            }
            n178 = local write "PSU Calc"(w578) -> ()
          }
          event Value Change {
            w828 = 1.0 ("x")
            w831 = 1000000.0 ("y")
            n179 = event-data() -> ()  [unwired: 1 in, 5 out]
            n180 = local read "PSU Calc"() -> (w837:T1)
            n181 = Unbundle By Name(w837) -> ("Window (Delta-T)"=w819:dbl, "Lower Cutoff"=w820:dbl, "Multiplier"=w822:u16, "Low Charge (fC)"=w812:dbl, "High Charge (fC)"=w811:dbl, "Low Mass (kg)"=w808:dbl, "High Mass (kg)"=w807:dbl, "Low Radius (µm)"=w806:dbl, "High Radius (µm)"=w805:dbl, "Exp. Voltage (MV)"=w788:dbl)
            n182 = Equal To 0?(x=w822) -> (x = 0?=w823:bool)
            n183 = Multiply(x=w788, y=1000000.0) -> (x*y=w787:dbl)
            n184 = Build Array(w806, w805) -> (w803:dbl[])
            n185 = Build Array(w808, w807) -> (w804:dbl[])
            n186 = Select(t=10.0, s=w823, f=1.0) -> (s? t:f=w821:dbl)
            n187 = Divide(x=w819, y=w821) -> (x/y=w834:dbl)
            n188 = Divide(x=w820, y=w821) -> (x/y=w832:dbl)
            n189 = Divide(x=w834, y=w831) -> (x/y=w826:dbl)
            n190 = Divide(x=w832, y=w831) -> (x/y=w829:dbl)
            n191 = Divide(x=w826, y=0.6) -> (x/y=w825:dbl)
            n192 = Divide(x=w829, y=0.6) -> (x/y=w827:dbl)
            n193 = Divide(x=w828, y=w827) -> (x/y=w814:dbl)
            n194 = Add(x=w825, y=w827) -> (x+y=w824:dbl)
            n195 = Divide(x=w828, y=w824) -> (x/y=w815:dbl)
            n196 = Build Array(w812, w811) -> (w810:dbl[])
            n197 = Build Array(w815, w814) -> (w813:dbl[])
            n198 = case shown="\"Charge\"" w816 {
              tunnel: w813 -> [w847 w894 w913]
              tunnel: w787 -> [w839 w900 w918]
              tunnel: w810 -> [w845 w893 _]
              tunnel: w809 -> [w838 w899 _]
              tunnel: w804 -> [w843 _ w911]
              tunnel: w803 -> [w841 _ w912]
              tunnel: [w846 w894 w913] -> w790
              tunnel: [w844 w893 w909] -> w800
              tunnel: [w842 w887 w911] -> w799
              tunnel: [w840 w889 w912] -> w798
              tunnel: w785 -> [w848 _ _]
              frame "Velocity" {
                n199 = case shown="\"Charge\"" w848 {
                  tunnel: w847 -> [w852 w856 w877]
                  tunnel: [w852 w856 w877] -> w846
                  tunnel: w845 -> [w851 w855 _]
                  tunnel: [w851 w855 w876] -> w844
                  tunnel: w843 -> [w850 _ w875]
                  tunnel: [w850 w857 w875] -> w842
                  tunnel: w841 -> [w849 _ w878]
                  tunnel: [w849 w854 w878] -> w840
                  tunnel: w839 -> [_ w859 w874]
                  tunnel: w838 -> [_ w858 _]
                  frame "Velocity" {
                  }
                  frame "Charge" {
                    n200 = Reverse 1D Array(array=w856) -> (reversed array=w853:dbl[])
                    n201 = Multiply(x=w855, y=2e-15 ("x")) -> (x*y=w861:dbl[])
                    n202 = Square(x=w853) -> (x^2=w863:dbl[])
                    n203 = Multiply(x=w861, y=w859) -> (x*y=w862:dbl[])
                    n204 = Divide(x=w862, y=w863) -> (x/y=w857:dbl[])
                    n205 = Multiply(x=w857, y=3.0 ("x")) -> (x*y=w865:dbl[])
                    n206 = Divide(x=w865, y=4.0 ("x")) -> (x/y=w866:dbl[])
                    n207 = Divide(x=w866, y=3.141592653589793) -> (x/y=w867:dbl[])
                    n208 = Divide(x=w867, y=w858) -> (x/y=w868:dbl[])
                    n209 = Y-th Root of X(1:w868, 2:3.0 ("x")) -> (0:w872:dbl[])
                    n210 = Multiply(x=w872, y=1000000.0 ("x")) -> (x*y=w854:dbl[])
                  }
                  frame "Mass" {
                    n211 = Square(x=w877) -> (x^2=w882:dbl[])
                    n212 = Divide(x=w875, y=2.0 ("x")) -> (x/y=w883:dbl[])
                    n213 = Multiply(x=w882, y=w883) -> (x*y=w881:dbl[])
                    n214 = Divide(x=w881, y=w874) -> (x/y=w880:dbl[])
                    n215 = Multiply(x=1000000000000000.0, y=w880) -> (x*y=w876:dbl[])
                  }
                }
              }
              frame "Charge" {
                n216 = Multiply(x=1e-15 ("Exp. Voltage (V)"), y=w893) -> (x*y=w891:dbl[])
                n217 = Multiply(x=w891, y=w900) -> (x*y=w898:dbl[])
                n218 = Reverse 1D Array(array=w894) -> (reversed array=w885:dbl[])
                n219 = Multiply(x=w898, y=2.0 ("Exp. Voltage (V)")) -> (x*y=w896:dbl[])
                n220 = Square(x=w885) -> (x^2=w895:dbl[])
                n221 = Divide(x=w896, y=w895) -> (x/y=w887:dbl[])
                n222 = Multiply(x=w887, y=3.0 ("Exp. Voltage (V)")) -> (x*y=w905:dbl[])
                n223 = local write "Variable 2"(enum32{"Velocity", "Charge", "Mass"}."Velocity" ("Variable 2")) -> ()
                n224 = Divide(x=w905, y=4.0 ("Exp. Voltage (V)")) -> (x/y=w903:dbl[])
                n225 = Divide(x=w903, y=3.141592653589793) -> (x/y=w901:dbl[])
                n226 = Divide(x=w901, y=w899) -> (x/y=w892:dbl[])
                n227 = Multiply(x=w892, y=1000000.0 ("Exp. Voltage (V)")) -> (x*y=w889:dbl[])
              }
              frame "Mass" {
                n228 = Divide(x=w911, y=w918) -> (x/y=w917:dbl[])
                n229 = Square(x=w913) -> (x^2=w914:dbl[])
                n230 = Divide(x=w917, y=2.0 ("Exp. Voltage (V)")) -> (x/y=w915:dbl[])
                n231 = Multiply(x=w915, y=w914) -> (x*y=w910:dbl[])
                n232 = Multiply(x=w910, y=1000000000000000.0 ("Exp. Voltage (V)")) -> (x*y=w909:dbl[])
                n233 = local write "Variable 2"(enum32{"Velocity", "Charge", "Mass"}."Velocity" ("Variable 2")) -> ()
              }
            }
            n234 = Divide(x=w790, y=1000.0 ("Exp. Voltage (V)")) -> (x/y=w791:dbl[])
            n235 = Index Array(array=w798) -> (element #1=w793:dbl, element #2=w792:dbl)  [unwired: 2 in]
            n236 = Index Array(array=w800) -> (element #1=w797:dbl, element #2=w796:dbl)  [unwired: 2 in]
            n237 = Index Array(array=w799) -> (element #1=w795:dbl, element #2=w794:dbl)  [unwired: 2 in]
            n238 = Index Array(array=w791) -> (element #1=w802:dbl, element #2=w801:dbl)  [unwired: 2 in]
            n239 = Bundle By Name(cluster=w837, "Low speed (km/s)"=w802, "High speed (km/s)"=w801, "Window (Delta-T)"=w819, "Lower Cutoff"=w820, "Multiplier"=w822, "Low Charge (fC)"=w797, "High Charge (fC)"=w796, "Low Mass (kg)"=w795, "High Mass (kg)"=w794, "Low Radius (µm)"=w793, "High Radius (µm)"=w792, "Exp. Voltage (MV)"=w788) -> (w836:T1)
            n240 = local write "PSU Calc"(w836) -> ()
          }
          event Value Change {
            n241 = event-data() -> ()  [unwired: 1 in, 5 out]
            n242 = local read "PSU Calc"() -> (w956:T1)
            n243 = Unbundle By Name(w956) -> ("Low speed (km/s)"=w955:dbl, "High speed (km/s)"=w954:dbl, "Window (Delta-T)"=w942:dbl, "Lower Cutoff"=w941:dbl, "Multiplier"=w940:u16, "Low Charge (fC)"=w952:dbl, "High Charge (fC)"=w951:dbl, "Low Mass (kg)"=w950:dbl, "High Mass (kg)"=w949:dbl, "Low Radius (µm)"=w948:dbl, "High Radius (µm)"=w947:dbl, "Exp. Voltage (MV)"=w922:dbl)
            n244 = Build Array(w948, w947) -> (w944:dbl[])
            n245 = Build Array(w955, w954) -> (w953:dbl[])
            n246 = Build Array(w952, w951) -> (w946:dbl[])
            n247 = Build Array(w950, w949) -> (w945:dbl[])
            n248 = Multiply(x=1000000.0, y=w922) -> (x*y=w921:dbl)
            n249 = case shown="\"Mass\"" w924 {
              tunnel: w953 -> [w967 w1002 _]
              tunnel: w921 -> [w980 w988 w1085]
              tunnel: w946 -> [w974 w994 w1088]
              tunnel: w943 -> [w979 w987 _]
              tunnel: w945 -> [_ w992 w1083]
              tunnel: w944 -> [_ w990 w1111]
              tunnel: [w967 w1001 w1078] -> w935
              tunnel: [w974 w993 w1088] -> w934
              tunnel: [w968 w991 w1083] -> w933
              tunnel: [w970 w989 w1111] -> w932
              tunnel: w942 -> [w966 w1000 _]
              tunnel: w941 -> [w965 w998 _]
              tunnel: w940 -> [w964 w996 _]
              tunnel: [w966 w999 w1091] -> w939
              tunnel: [w965 w997 w1090] -> w938
              tunnel: [w964 w995 w1089] -> w937
              tunnel: w919 -> [_ w1003 _]
              frame "Velocity" {
                n250 = Multiply(x=1e-15 ("Exp. Voltage (V)"), y=w974) -> (x*y=w972:dbl[])
                n251 = Multiply(x=w972, y=w980) -> (x*y=w978:dbl[])
                n252 = Multiply(x=w967, y=1000.0 ("Exp. Voltage (V)")) -> (x*y=w962:dbl[])
                n253 = Reverse 1D Array(array=w962) -> (reversed array=w958:dbl[])
                n254 = Square(x=w958) -> (x^2=w975:dbl[])
                n255 = Multiply(x=w978, y=2.0 ("Exp. Voltage (V)")) -> (x*y=w976:dbl[])
                n256 = Divide(x=w976, y=w975) -> (x/y=w968:dbl[])
                n257 = Multiply(x=w968, y=3.0 ("Exp. Voltage (V)")) -> (x*y=w985:dbl[])
                n258 = Divide(x=w985, y=4.0 ("Exp. Voltage (V)")) -> (x/y=w983:dbl[])
                n259 = Divide(x=w983, y=3.141592653589793) -> (x/y=w981:dbl[])
                n260 = local write "Variable 2"(enum32{"Velocity", "Charge", "Mass"}."Charge" ("Variable 2")) -> ()
                n261 = Divide(x=w981, y=w979) -> (x/y=w973:dbl[])
                n262 = Y-th Root of X(1:w973, 2:3.0 ("Exp. Voltage (V)")) -> (0:w960:dbl[])
                n263 = Multiply(x=w960, y=1000000.0 ("Exp. Voltage (V)")) -> (x*y=w970:dbl[])
              }
              frame "Charge" {
                n264 = case shown="\"Velocity\"" w1003 {
                  tunnel: w1002 -> [w1007 w1038 _]
                  tunnel: [w1007 w1038 w1042] -> w1001
                  tunnel: w1000 -> [w1031 w1037 _]
                  tunnel: [w1031 w1037 w1055] -> w999
                  tunnel: w998 -> [w1030 w1036 _]
                  tunnel: [w1030 w1036 w1054] -> w997
                  tunnel: w996 -> [w1029 w1035 _]
                  tunnel: [w1029 w1035 w1053] -> w995
                  tunnel: w994 -> [w1012 w1034 w1040]
                  tunnel: [w1012 w1034 w1040] -> w993
                  tunnel: w992 -> [_ w1033 w1041]
                  tunnel: [w1008 w1033 w1041] -> w991
                  tunnel: w990 -> [_ w1032 w1043]
                  tunnel: [w1009 w1032 w1043] -> w989
                  tunnel: w988 -> [w1011 _ w1045]
                  tunnel: w987 -> [w1010 _ _]
                  frame "Velocity" {
                    n265 = Multiply(x=1e-15 ("Exp. Voltage (V)"), y=w1012) -> (x*y=w1017:dbl[])
                    n266 = Multiply(x=w1017, y=w1011) -> (x*y=w1022:dbl[])
                    n267 = Multiply(x=w1007, y=1000.0 ("Exp. Voltage (V)")) -> (x*y=w1014:dbl[])
                    n268 = Reverse 1D Array(array=w1014) -> (reversed array=w1004:dbl[])
                    n269 = Square(x=w1004) -> (x^2=w1019:dbl[])
                    n270 = Multiply(x=w1022, y=2.0 ("Exp. Voltage (V)")) -> (x*y=w1020:dbl[])
                    n271 = Divide(x=w1020, y=w1019) -> (x/y=w1008:dbl[])
                    n272 = Multiply(x=w1008, y=3.0 ("Exp. Voltage (V)")) -> (x*y=w1027:dbl[])
                    n273 = Divide(x=w1027, y=4.0 ("Exp. Voltage (V)")) -> (x/y=w1025:dbl[])
                    n274 = Divide(x=w1025, y=3.141592653589793) -> (x/y=w1023:dbl[])
                    n275 = Divide(x=w1023, y=w1010) -> (x/y=w1018:dbl[])
                    n276 = Y-th Root of X(1:w1018, 2:3.0 ("Exp. Voltage (V)")) -> (0:w1006:dbl[])
                    n277 = Multiply(x=w1006, y=1000000.0 ("Exp. Voltage (V)")) -> (x*y=w1009:dbl[])
                  }
                  frame "Charge" {
                  }
                  frame "Mass" {
                    w1062 = 99.989
                    w1060 = 1000000.0 ("y")
                    n278 = Multiply(x=w1040, y=1e-15 ("x")) -> (x*y=w1051:dbl[])
                    n279 = Reverse 1D Array(array=w1041) -> (reversed array=w1039:dbl[])
                    n280 = Multiply(x=w1051, y=w1045) -> (x*y=w1050:dbl[])
                    n281 = Divide(x=w1050, y=w1039) -> (x/y=w1049:dbl[])
                    n282 = Multiply(x=w1049, y=2.0 ("x")) -> (x*y=w1047:dbl[])
                    n283 = Square Root(x=w1047) -> (sqrt(x)=w1044:dbl[])
                    n284 = Index Array(array=w1044) -> (element #1=w1073:dbl, element #2=w1074:dbl)  [unwired: 2 in]
                    n285 = Divide(x=0.6, y=w1073) -> (x/y=w1058:dbl)
                    n286 = Divide(x=0.6, y=w1074) -> (x/y=w1059:dbl)
                    n287 = Subtract(x=w1058, y=w1059) -> (x-y=w1061:dbl)
                    n288 = Multiply(x=w1059, y=w1060) -> (x*y=w1068:dbl)
                    n289 = Multiply(x=w1061, y=w1060) -> (x*y=w1067:dbl)
                    n290 = Less?(x=w1068, y=w1062) -> (x < y?=w1063:bool)
                    n291 = Less?(x=w1067, y=w1062) -> (x < y?=w1064:bool)
                    n292 = Divide(x=w1044, y=1000.0 ("x")) -> (x/y=w1042:dbl[])
                    n293 = And(x=w1063, y=w1064) -> (x .and. y?=w1070:bool)
                    n294 = Select(t=u16 0 ("Multiplier"), s=w1070, f=u16 1 ("Multiplier")) -> (s? t:f=w1053:u16)
                    n295 = Select(t=10.0, s=w1070, f=1.0) -> (s? t:f=w1069:dbl)
                    n296 = Multiply(x=w1067, y=w1069) -> (x*y=w1055:dbl)
                    n297 = Multiply(x=w1068, y=w1069) -> (x*y=w1054:dbl)
                  }
                }
              }
              frame "Mass" {
                w1098 = 99.989
                w1096 = 1000000.0 ("y")
                n298 = Multiply(x=w1088, y=1e-15 ("x")) -> (x*y=w1086:dbl[])
                n299 = Multiply(x=w1086, y=w1085) -> (x*y=w1084:dbl[])
                n300 = Reverse 1D Array(array=w1083) -> (reversed array=w1075:dbl[])
                n301 = Divide(x=w1084, y=w1075) -> (x/y=w1082:dbl[])
                n302 = Multiply(x=w1082, y=2.0 ("x")) -> (x*y=w1080:dbl[])
                n303 = Square Root(x=w1080) -> (sqrt(x)=w1077:dbl[])
                n304 = Index Array(array=w1077) -> (element #1=w1109:dbl, element #2=w1110:dbl)  [unwired: 2 in]
                n305 = Divide(x=0.6, y=w1109) -> (x/y=w1094:dbl)
                n306 = Divide(x=0.6, y=w1110) -> (x/y=w1095:dbl)
                n307 = Subtract(x=w1094, y=w1095) -> (x-y=w1097:dbl)
                n308 = Multiply(x=w1095, y=w1096) -> (x*y=w1104:dbl)
                n309 = Multiply(x=w1097, y=w1096) -> (x*y=w1103:dbl)
                n310 = Divide(x=w1077, y=1000.0 ("x")) -> (x/y=w1078:dbl[])
                n311 = Less?(x=w1104, y=w1098) -> (x < y?=w1099:bool)
                n312 = Less?(x=w1103, y=w1098) -> (x < y?=w1100:bool)
                n313 = local write "Variable 2"(enum32{"Velocity", "Charge", "Mass"}."Charge" ("Variable 2")) -> ()
                n314 = And(x=w1099, y=w1100) -> (x .and. y?=w1106:bool)
                n315 = Select(t=u16 0 ("Multiplier"), s=w1106, f=u16 1 ("Multiplier")) -> (s? t:f=w1089:u16)
                n316 = Select(t=10.0, s=w1106, f=1.0) -> (s? t:f=w1105:dbl)
                n317 = Multiply(x=w1103, y=w1105) -> (x*y=w1091:dbl)
                n318 = Multiply(x=w1104, y=w1105) -> (x*y=w1090:dbl)
              }
            }
            n319 = Index Array(array=w935) -> (element #1=w936:dbl, element #2=w929:dbl)  [unwired: 2 in]
            n320 = Index Array(array=w934) -> (element #1=w931:dbl, element #2=w930:dbl)  [unwired: 2 in]
            n321 = Index Array(array=w932) -> (element #1=w926:dbl, element #2=w925:dbl)  [unwired: 2 in]
            n322 = Index Array(array=w933) -> (element #1=w928:dbl, element #2=w927:dbl)  [unwired: 2 in]
            n323 = Bundle By Name(cluster=w956, "Low speed (km/s)"=w936, "High speed (km/s)"=w929, "Window (Delta-T)"=w939, "Lower Cutoff"=w938, "Multiplier"=w937, "Low Charge (fC)"=w931, "High Charge (fC)"=w930, "Low Mass (kg)"=w928, "High Mass (kg)"=w927, "Low Radius (µm)"=w926, "High Radius (µm)"=w925, "Exp. Voltage (MV)"=w922) -> (w957:T1)
            n324 = local write "PSU Calc"(w957) -> ()
          }
          event Value Change {
            n325 = event-data() -> ()  [unwired: 1 in, 5 out]
            n326 = local read "PSU Calc"() -> (w1149:T1)
            n327 = Unbundle By Name(w1149) -> ("Low speed (km/s)"=w1148:dbl, "High speed (km/s)"=w1147:dbl, "Window (Delta-T)"=w1135:dbl, "Lower Cutoff"=w1134:dbl, "Multiplier"=w1133:u16, "Low Charge (fC)"=w1145:dbl, "High Charge (fC)"=w1144:dbl, "Low Mass (kg)"=w1143:dbl, "High Mass (kg)"=w1142:dbl, "Low Radius (µm)"=w1141:dbl, "High Radius (µm)"=w1140:dbl, "Exp. Voltage (MV)"=w1114:dbl)
            n328 = Build Array(w1141, w1140) -> (w1137:dbl[])
            n329 = Build Array(w1148, w1147) -> (w1146:dbl[])
            n330 = Build Array(w1145, w1144) -> (w1139:dbl[])
            n331 = Build Array(w1143, w1142) -> (w1138:dbl[])
            n332 = Multiply(x=w1114, y=1000000.0) -> (x*y=w1113:dbl)
            n333 = case shown="\"Mass\"" w1116 {
              tunnel: w1146 -> [w1167 w1253 w1319]
              tunnel: w1139 -> [w1166 w1252 w1318]
              tunnel: w1138 -> [w1165 w1251 w1317]
              tunnel: w1137 -> [w1164 w1250 w1316]
              tunnel: w1113 -> [w1163 w1249 w1315]
              tunnel: w1136 -> [w1162 w1248 w1314]
              tunnel: w1135 -> [w1161 w1247 w1313]
              tunnel: w1134 -> [w1160 w1246 w1312]
              tunnel: w1133 -> [w1159 w1245 w1311]
              tunnel: [w1158 w1244 w1310] -> w1132
              tunnel: [w1157 w1243 w1309] -> w1131
              tunnel: [w1156 w1242 w1308] -> w1130
              tunnel: [w1155 w1241 w1307] -> w1128
              tunnel: [w1154 w1240 w1306] -> w1127
              tunnel: [w1153 w1239 w1305] -> w1126
              tunnel: [w1152 w1238 w1304] -> w1125
              tunnel: w1117 -> [w1151 w1237 w1303]
              frame "Charge" {
                n334 = case shown="\"Mass\"" w1151 {
                  tunnel: w1167 -> [w1174 w1200 _]
                  tunnel: w1163 -> [w1187 _ w1210]
                  tunnel: w1166 -> [w1181 w1199 w1213]
                  tunnel: w1162 -> [w1186 _ _]
                  tunnel: w1165 -> [_ w1198 w1208]
                  tunnel: w1164 -> [_ w1197 w1236]
                  tunnel: [w1174 w1200 w1204] -> w1155
                  tunnel: [w1181 w1199 w1213] -> w1154
                  tunnel: [w1175 w1198 w1208] -> w1153
                  tunnel: [w1177 w1197 w1236] -> w1152
                  tunnel: w1161 -> [w1173 w1196 _]
                  tunnel: w1160 -> [w1172 w1195 _]
                  tunnel: w1159 -> [w1171 w1194 _]
                  tunnel: [w1173 w1196 w1216] -> w1158
                  tunnel: [w1172 w1195 w1215] -> w1157
                  tunnel: [w1171 w1194 w1214] -> w1156
                  frame "Velocity" {
                    n335 = Multiply(x=1e-15 ("Exp. Voltage (V)"), y=w1181) -> (x*y=w1179:dbl[])
                    n336 = Multiply(x=w1179, y=w1187) -> (x*y=w1185:dbl[])
                    n337 = Multiply(x=w1174, y=1000.0 ("Exp. Voltage (V)")) -> (x*y=w1170:dbl[])
                    n338 = Reverse 1D Array(array=w1170) -> (reversed array=w1168:dbl[])
                    n339 = Square(x=w1168) -> (x^2=w1182:dbl[])
                    n340 = Multiply(x=w1185, y=2.0 ("Exp. Voltage (V)")) -> (x*y=w1183:dbl[])
                    n341 = Divide(x=w1183, y=w1182) -> (x/y=w1175:dbl[])
                    n342 = Multiply(x=w1175, y=3.0 ("Exp. Voltage (V)")) -> (x*y=w1192:dbl[])
                    n343 = Divide(x=w1192, y=4.0 ("Exp. Voltage (V)")) -> (x/y=w1190:dbl[])
                    n344 = Divide(x=w1190, y=3.141592653589793) -> (x/y=w1188:dbl[])
                    n345 = Divide(x=w1188, y=w1186) -> (x/y=w1180:dbl[])
                    n346 = Multiply(x=w1180, y=1000000.0 ("Exp. Voltage (V)")) -> (x*y=w1177:dbl[])
                  }
                  frame "Charge" {
                  }
                  frame "Mass" {
                    w1223 = 99.989
                    w1221 = 1000000.0 ("y")
                    n347 = Multiply(x=w1213, y=1e-15 ("x")) -> (x*y=w1211:dbl[])
                    n348 = Multiply(x=w1211, y=w1210) -> (x*y=w1209:dbl[])
                    n349 = Reverse 1D Array(array=w1208) -> (reversed array=w1201:dbl[])
                    n350 = Divide(x=w1209, y=w1201) -> (x/y=w1207:dbl[])
                    n351 = Multiply(x=w1207, y=2.0 ("x")) -> (x*y=w1205:dbl[])
                    n352 = Square Root(x=w1205) -> (sqrt(x)=w1203:dbl[])
                    n353 = Index Array(array=w1203) -> (element #1=w1234:dbl, element #2=w1235:dbl)  [unwired: 2 in]
                    n354 = Divide(x=0.6, y=w1234) -> (x/y=w1219:dbl)
                    n355 = Divide(x=0.6, y=w1235) -> (x/y=w1220:dbl)
                    n356 = Subtract(x=w1219, y=w1220) -> (x-y=w1222:dbl)
                    n357 = Multiply(x=w1220, y=w1221) -> (x*y=w1229:dbl)
                    n358 = Multiply(x=w1222, y=w1221) -> (x*y=w1228:dbl)
                    n359 = Divide(x=w1203, y=1000.0 ("x")) -> (x/y=w1204:dbl[])
                    n360 = Less?(x=w1229, y=w1223) -> (x < y?=w1224:bool)
                    n361 = Less?(x=w1228, y=w1223) -> (x < y?=w1225:bool)
                    n362 = And(x=w1224, y=w1225) -> (x .and. y?=w1231:bool)
                    n363 = Select(t=u16 0 ("Multiplier"), s=w1231, f=u16 1 ("Multiplier")) -> (s? t:f=w1214:u16)
                    n364 = Select(t=10.0, s=w1231, f=1.0) -> (s? t:f=w1230:dbl)
                    n365 = Multiply(x=w1228, y=w1230) -> (x*y=w1216:dbl)
                    n366 = Multiply(x=w1229, y=w1230) -> (x*y=w1215:dbl)
                  }
                }
              }
              frame "Velocity" {
                n367 = case shown="\"Charge\"" w1237 {
                  tunnel: w1253 -> [w1260 w1267 w1292]
                  tunnel: w1249 -> [_ w1280 w1290]
                  tunnel: w1252 -> [w1259 w1274 _]
                  tunnel: w1248 -> [_ w1279 _]
                  tunnel: w1251 -> [w1258 _ w1291]
                  tunnel: w1250 -> [w1257 _ w1299]
                  tunnel: [w1260 w1267 w1292] -> w1241
                  tunnel: [w1259 w1274 w1289] -> w1240
                  tunnel: [w1258 w1268 w1291] -> w1239
                  tunnel: [w1257 w1270 w1299] -> w1238
                  tunnel: w1247 -> [w1256 w1266 w1302]
                  tunnel: w1246 -> [w1255 w1265 w1301]
                  tunnel: w1245 -> [w1254 w1264 w1300]
                  tunnel: [w1256 w1266 w1302] -> w1244
                  tunnel: [w1255 w1265 w1301] -> w1243
                  tunnel: [w1254 w1264 w1300] -> w1242
                  frame "Velocity" {
                  }
                  frame "Charge" {
                    n368 = Multiply(x=1e-15 ("Exp. Voltage (V)"), y=w1274) -> (x*y=w1272:dbl[])
                    n369 = Multiply(x=w1272, y=w1280) -> (x*y=w1278:dbl[])
                    n370 = Multiply(x=w1267, y=1000.0 ("Exp. Voltage (V)")) -> (x*y=w1263:dbl[])
                    n371 = Reverse 1D Array(array=w1263) -> (reversed array=w1261:dbl[])
                    n372 = Square(x=w1261) -> (x^2=w1275:dbl[])
                    n373 = Multiply(x=w1278, y=2.0 ("Exp. Voltage (V)")) -> (x*y=w1276:dbl[])
                    n374 = Divide(x=w1276, y=w1275) -> (x/y=w1268:dbl[])
                    n375 = Multiply(x=w1268, y=3.0 ("Exp. Voltage (V)")) -> (x*y=w1285:dbl[])
                    n376 = Divide(x=w1285, y=4.0 ("Exp. Voltage (V)")) -> (x/y=w1283:dbl[])
                    n377 = Divide(x=w1283, y=3.141592653589793) -> (x/y=w1281:dbl[])
                    n378 = Divide(x=w1281, y=w1279) -> (x/y=w1273:dbl[])
                    n379 = Multiply(x=w1273, y=1000000.0 ("Exp. Voltage (V)")) -> (x*y=w1270:dbl[])
                  }
                  frame "Mass" {
                    n380 = Divide(x=w1291, y=w1290) -> (x/y=w1298:dbl[])
                    n381 = Multiply(x=w1292, y=1000.0 ("Exp. Voltage (V)")) -> (x*y=w1288:dbl[])
                    n382 = Square(x=w1288) -> (x^2=w1295:dbl[])
                    n383 = Divide(x=w1298, y=2.0 ("Exp. Voltage (V)")) -> (x/y=w1296:dbl[])
                    n384 = Multiply(x=w1296, y=w1295) -> (x*y=w1294:dbl[])
                    n385 = Multiply(x=w1294, y=1000000000000000.0 ("Exp. Voltage (V)")) -> (x*y=w1289:dbl[])
                  }
                }
              }
              frame "Mass" {
                n386 = case shown="\"Velocity\"" w1303 {
                  tunnel: w1319 -> [w1325 _ w1378]
                  tunnel: w1315 -> [w1329 w1342 _]
                  tunnel: w1318 -> [_ w1343 w1377]
                  tunnel: w1314 -> [_ _ _]
                  tunnel: w1317 -> [w1326 w1346 w1376]
                  tunnel: w1316 -> [w1327 w1345 w1375]
                  tunnel: [w1325 w1338 w1378] -> w1307
                  tunnel: [w1321 w1343 w1377] -> w1306
                  tunnel: [w1326 w1346 w1376] -> w1305
                  tunnel: [w1327 w1345 w1375] -> w1304
                  tunnel: w1313 -> [w1324 _ w1374]
                  tunnel: w1312 -> [w1323 _ w1373]
                  tunnel: w1311 -> [w1322 _ w1372]
                  tunnel: [w1324 w1339 w1374] -> w1310
                  tunnel: [w1323 w1340 w1373] -> w1309
                  tunnel: [w1322 w1341 w1372] -> w1308
                  frame "Velocity" {
                    n387 = Multiply(x=w1325, y=1000.0 ("Lower Cutoff")) -> (x*y=w1332:dbl[])
                    n388 = Divide(x=w1326, y=2.0 ("Lower Cutoff")) -> (x/y=w1333:dbl[])
                    n389 = Square(x=w1332) -> (x^2=w1334:dbl[])
                    n390 = Multiply(x=w1334, y=w1333) -> (x*y=w1330:dbl[])
                    n391 = Divide(x=w1330, y=w1329) -> (x/y=w1328:dbl[])
                    n392 = Multiply(x=w1328, y=1000000000000000.0 ("Lower Cutoff")) -> (x*y=w1321:dbl[])
                  }
                  frame "Charge" {
                    w1359 = 99.989
                    w1357 = 1000000.0 ("y")
                    n393 = Multiply(x=w1343, y=1e-15 ("x")) -> (x*y=w1351:dbl[])
                    n394 = Multiply(x=w1351, y=w1342) -> (x*y=w1350:dbl[])
                    n395 = Reverse 1D Array(array=w1346) -> (reversed array=w1336:dbl[])
                    n396 = Divide(x=w1350, y=w1336) -> (x/y=w1349:dbl[])
                    n397 = Multiply(x=w1349, y=2.0 ("x")) -> (x*y=w1347:dbl[])
                    n398 = Square Root(x=w1347) -> (sqrt(x)=w1344:dbl[])
                    n399 = Index Array(array=w1344) -> (element #1=w1370:dbl, element #2=w1371:dbl)  [unwired: 2 in]
                    n400 = Divide(x=0.6, y=w1370) -> (x/y=w1355:dbl)
                    n401 = Divide(x=0.6, y=w1371) -> (x/y=w1356:dbl)
                    n402 = Subtract(x=w1355, y=w1356) -> (x-y=w1358:dbl)
                    n403 = Multiply(x=w1356, y=w1357) -> (x*y=w1365:dbl)
                    n404 = Multiply(x=w1358, y=w1357) -> (x*y=w1364:dbl)
                    n405 = Less?(x=w1365, y=w1359) -> (x < y?=w1360:bool)
                    n406 = Less?(x=w1364, y=w1359) -> (x < y?=w1361:bool)
                    n407 = Divide(x=w1344, y=1000.0 ("x")) -> (x/y=w1338:dbl[])
                    n408 = And(x=w1360, y=w1361) -> (x .and. y?=w1367:bool)
                    n409 = Select(t=u16 0 ("Multiplier"), s=w1367, f=u16 1 ("Multiplier")) -> (s? t:f=w1341:u16)
                    n410 = Select(t=10.0, s=w1367, f=1.0) -> (s? t:f=w1366:dbl)
                    n411 = Multiply(x=w1364, y=w1366) -> (x*y=w1339:dbl)
                    n412 = Multiply(x=w1365, y=w1366) -> (x*y=w1340:dbl)
                  }
                  frame "Mass" {
                  }
                }
              }
            }
            n413 = Index Array(array=w1128) -> (element #1=w1129:dbl, element #2=w1122:dbl)  [unwired: 2 in]
            n414 = Index Array(array=w1127) -> (element #1=w1124:dbl, element #2=w1123:dbl)  [unwired: 2 in]
            n415 = Index Array(array=w1125) -> (element #1=w1119:dbl, element #2=w1118:dbl)  [unwired: 2 in]
            n416 = Index Array(array=w1126) -> (element #1=w1121:dbl, element #2=w1120:dbl)  [unwired: 2 in]
            n417 = Bundle By Name(cluster=w1149, "Low speed (km/s)"=w1129, "High speed (km/s)"=w1122, "Window (Delta-T)"=w1132, "Lower Cutoff"=w1131, "Multiplier"=w1130, "Low Charge (fC)"=w1124, "High Charge (fC)"=w1123, "Low Mass (kg)"=w1121, "High Mass (kg)"=w1120, "Low Radius (µm)"=w1119, "High Radius (µm)"=w1118, "Exp. Voltage (MV)"=w1114) -> (w1150:T1)
            n418 = local write "PSU Calc"(w1150) -> ()
          }
          event "Variable 1": Value Change {
            n419 = event-data() -> ("OldVal"=w1384:enum32{"Velocity", "Charge", "Mass"}, "NewVal"=w1386:enum32{"Velocity", "Charge", "Mass"})  [unwired: 1 in, 3 out]
            n420 = property on="Variable 2" class="RadioBtnsControl (strict)"(error in=w1387) -> (error out=w1388:errorcluster, "Controls[]"=w1393:refnum<vi>[])  [unwired: 1 in, 1 out]
            n421 = Index Array(array=w1393, index=w1384) -> (element=w1392:refnum<vi>)
            n422 = Index Array(array=w1393, index=w1386) -> (element=w1391:refnum<vi>)
            n423 = property class="Ctl"(reference=w1392, error in=w1388, "DisabledEnum"=T4."Enabled" ("Disabled")) -> (error out=w1381:errorcluster)  [unwired: 1 out]
            n424 = property class="Ctl"(reference=w1391, error in=w1388, "DisabledEnum"=T4."Disabled and Grayed Out" ("Disabled")) -> (error out=w1380:errorcluster)  [unwired: 1 out]
            n425 = Equal?(x=w1386, y=w1383) -> (x = y?=w1385:bool)
            n426 = Select(t=w1384, s=w1385, f=w1383) -> (s? t:f=w1382:enum32{"Velocity", "Charge", "Mass"})
            n427 = Merge Errors(w1381, w1380) -> (w1379:errorcluster)
            n428 = local write "Variable 2"(w1382) -> ()
          }
          event Value Change {
            n429 = event-data() -> ()  [unwired: 1 in, 5 out]
            n430 = local read "PSU Calc"() -> (w1438:T1)
            n431 = Unbundle By Name(w1438) -> ("Low speed (km/s)"=w1437:dbl, "High speed (km/s)"=w1436:dbl, "Window (Delta-T)"=w1429:dbl, "Lower Cutoff"=w1428:dbl, "Multiplier"=w1427:u16, "Low Charge (fC)"=w1434:dbl, "High Charge (fC)"=w1433:dbl, "Low Mass (kg)"=w1432:dbl, "High Mass (kg)"=w1431:dbl, "Exp. Voltage (MV)"=w1397:dbl)  [unwired: 2 out]
            n432 = Build Array(w1437, w1436) -> (w1435:dbl[])
            n433 = Build Array(w1434, w1433) -> (w1430:dbl[])
            n434 = Build Array(w1432, w1431) -> (w1411:dbl[])
            n435 = Multiply(x=1000000.0, y=w1397) -> (x*y=w1396:dbl)
            n436 = Multiply(x=w1411, y=3.0 ("x")) -> (x*y=w1409:dbl[])
            n437 = Divide(x=w1409, y=4.0 ("x")) -> (x/y=w1407:dbl[])
            n438 = case shown="\"Velocity\"" w1412 {
              tunnel: w1435 -> [w1449 _ w1504]
              tunnel: w1396 -> [w1443 w1466 w1492]
              tunnel: w1430 -> [_ w1469 w1496]
              tunnel: w1411 -> [w1451 w1464 w1493]
              tunnel: [w1449 w1459 w1503] -> w1422
              tunnel: [w1441 w1469 w1495] -> w1421
              tunnel: [w1451 w1464 w1494] -> w1420
              tunnel: w1429 -> [w1455 _ w1502]
              tunnel: w1428 -> [w1454 _ w1500]
              tunnel: w1427 -> [w1453 _ w1498]
              tunnel: [w1455 w1472 w1501] -> w1426
              tunnel: [w1454 w1471 w1499] -> w1425
              tunnel: [w1453 w1470 w1497] -> w1424
              tunnel: w1394 -> [_ _ w1505]
              frame "Velocity" {
                n439 = Multiply(x=w1449, y=1000.0 ("Lower Cutoff")) -> (x*y=w1446:dbl[])
                n440 = Divide(x=w1451, y=2.0 ("Lower Cutoff")) -> (x/y=w1447:dbl[])
                n441 = Square(x=w1446) -> (x^2=w1448:dbl[])
                n442 = Multiply(x=w1448, y=w1447) -> (x*y=w1444:dbl[])
                n443 = Divide(x=w1444, y=w1443) -> (x/y=w1442:dbl[])
                n444 = Multiply(x=1000000000000000.0 ("Lower Cutoff"), y=w1442) -> (x*y=w1441:dbl[])
                n445 = local write "Variable 2"(enum32{"Velocity", "Charge", "Mass"}."Mass" ("Variable 2")) -> ()
              }
              frame "Charge" {
                w1479 = 99.989
                w1477 = 1000000.0 ("y")
                n446 = Multiply(x=w1469, y=1e-15 ("x")) -> (x*y=w1467:dbl[])
                n447 = Multiply(x=w1467, y=w1466) -> (x*y=w1465:dbl[])
                n448 = Reverse 1D Array(array=w1464) -> (reversed array=w1456:dbl[])
                n449 = Divide(x=w1465, y=w1456) -> (x/y=w1463:dbl[])
                n450 = Multiply(x=w1463, y=2.0 ("x")) -> (x*y=w1461:dbl[])
                n451 = Square Root(x=w1461) -> (sqrt(x)=w1458:dbl[])
                n452 = Index Array(array=w1458) -> (element #1=w1490:dbl, element #2=w1491:dbl)  [unwired: 2 in]
                n453 = Divide(x=0.6, y=w1490) -> (x/y=w1475:dbl)
                n454 = Divide(x=0.6, y=w1491) -> (x/y=w1476:dbl)
                n455 = Subtract(x=w1475, y=w1476) -> (x-y=w1478:dbl)
                n456 = Multiply(x=w1476, y=w1477) -> (x*y=w1485:dbl)
                n457 = Multiply(x=w1478, y=w1477) -> (x*y=w1484:dbl)
                n458 = Divide(x=w1458, y=1000.0) -> (x/y=w1459:dbl[])
                n459 = Less?(x=w1485, y=w1479) -> (x < y?=w1480:bool)
                n460 = Less?(x=w1484, y=w1479) -> (x < y?=w1481:bool)
                n461 = local write "Variable 2"(enum32{"Velocity", "Charge", "Mass"}."Mass" ("Variable 2")) -> ()
                n462 = And(x=w1480, y=w1481) -> (x .and. y?=w1487:bool)
                n463 = Select(t=u16 0 ("Multiplier"), s=w1487, f=u16 1 ("Multiplier")) -> (s? t:f=w1470:u16)
                n464 = Select(t=10.0, s=w1487, f=1.0) -> (s? t:f=w1486:dbl)
                n465 = Multiply(x=w1484, y=w1486) -> (x*y=w1472:dbl)
                n466 = Multiply(x=w1485, y=w1486) -> (x*y=w1471:dbl)
              }
              frame "Mass" {
                n467 = case shown="\"Charge\"" w1505 {
                  tunnel: w1504 -> [w1508 _ w1561]
                  tunnel: [w1508 w1522 w1561] -> w1503
                  tunnel: w1502 -> [w1512 _ w1560]
                  tunnel: [w1512 w1536 w1560] -> w1501
                  tunnel: w1500 -> [w1511 _ w1559]
                  tunnel: [w1511 w1535 w1559] -> w1499
                  tunnel: w1498 -> [w1510 _ w1558]
                  tunnel: [w1510 w1534 w1558] -> w1497
                  tunnel: w1496 -> [_ w1525 w1557]
                  tunnel: [w1513 w1525 w1557] -> w1495
                  tunnel: [w1506 w1523 w1556] -> w1494
                  tunnel: w1493 -> [w1506 w1523 w1556]
                  tunnel: w1492 -> [w1514 w1524 _]
                  frame "Velocity" {
                    n468 = Multiply(x=w1508, y=1000.0 ("x")) -> (x*y=w1509:dbl[])
                    n469 = Square(x=w1509) -> (x^2=w1518:dbl[])
                    n470 = Divide(x=w1506, y=2.0 ("x")) -> (x/y=w1519:dbl[])
                    n471 = Multiply(x=w1518, y=w1519) -> (x*y=w1517:dbl[])
                    n472 = Divide(x=w1517, y=w1514) -> (x/y=w1516:dbl[])
                    n473 = Multiply(x=1000000000000000.0, y=w1516) -> (x*y=w1513:dbl[])
                  }
                  frame "Charge" {
                    w1549 = 99.989
                    w1551 = 1000000.0 ("y")
                    n474 = Multiply(x=w1525, y=1e-15 ("x")) -> (x*y=w1532:dbl[])
                    n475 = Multiply(x=w1532, y=w1524) -> (x*y=w1531:dbl[])
                    n476 = Reverse 1D Array(array=w1523) -> (reversed array=w1521:dbl[])
                    n477 = Divide(x=w1531, y=w1521) -> (x/y=w1530:dbl[])
                    n478 = Multiply(x=w1530, y=2.0 ("x")) -> (x*y=w1528:dbl[])
                    n479 = Square Root(x=w1528) -> (sqrt(x)=w1526:dbl[])
                    n480 = Index Array(array=w1526) -> (element #1=w1538:dbl, element #2=w1537:dbl)  [unwired: 2 in]
                    n481 = Divide(x=0.6, y=w1538) -> (x/y=w1553:dbl)
                    n482 = Divide(x=0.6, y=w1537) -> (x/y=w1552:dbl)
                    n483 = Subtract(x=w1553, y=w1552) -> (x-y=w1550:dbl)
                    n484 = Multiply(x=w1552, y=w1551) -> (x*y=w1543:dbl)
                    n485 = Multiply(x=w1550, y=w1551) -> (x*y=w1544:dbl)
                    n486 = Less?(x=w1543, y=w1549) -> (x < y?=w1548:bool)
                    n487 = Less?(x=w1544, y=w1549) -> (x < y?=w1547:bool)
                    n488 = Divide(x=w1526, y=1000.0 ("x")) -> (x/y=w1522:dbl[])
                    n489 = And(x=w1548, y=w1547) -> (x .and. y?=w1541:bool)
                    n490 = Select(t=u16 0 ("Multiplier"), s=w1541, f=u16 1 ("Multiplier")) -> (s? t:f=w1534:u16)
                    n491 = Select(t=10.0, s=w1541, f=1.0) -> (s? t:f=w1542:dbl)
                    n492 = Multiply(x=w1544, y=w1542) -> (x*y=w1536:dbl)
                    n493 = Multiply(x=w1543, y=w1542) -> (x*y=w1535:dbl)
                  }
                  frame "Mass" {
                  }
                }
              }
            }
            n494 = Divide(x=w1407, y=3.141592653589793) -> (x/y=w1405:dbl[])
            n495 = Divide(x=w1405, y=w1404) -> (x/y=w1403:dbl[])
            n496 = Y-th Root of X(1:w1403, 2:3.0 ("x")) -> (0:w1401:dbl[])
            n497 = Multiply(x=w1401, y=1000000.0 ("x")) -> (x*y=w1399:dbl[])
            n498 = Index Array(array=w1422) -> (element #1=w1423:dbl, element #2=w1417:dbl)  [unwired: 2 in]
            n499 = Index Array(array=w1421) -> (element #1=w1419:dbl, element #2=w1418:dbl)  [unwired: 2 in]
            n500 = Index Array(array=w1399) -> (element #1=w1414:dbl, element #2=w1413:dbl)  [unwired: 2 in]
            n501 = Index Array(array=w1420) -> (element #1=w1416:dbl, element #2=w1415:dbl)  [unwired: 2 in]
            n502 = Bundle By Name(cluster=w1438, "Low speed (km/s)"=w1423, "High speed (km/s)"=w1417, "Window (Delta-T)"=w1426, "Lower Cutoff"=w1425, "Multiplier"=w1424, "Low Charge (fC)"=w1419, "High Charge (fC)"=w1418, "Low Mass (kg)"=w1416, "High Mass (kg)"=w1415, "Low Radius (µm)"=w1414, "High Radius (µm)"=w1413, "Exp. Voltage (MV)"=w1397) -> (w1439:T1)
            n503 = local write "PSU Calc"(w1439) -> ()
          }
          event Value Change {
            n504 = event-data() -> ()  [unwired: 1 in, 5 out]
            n505 = local read "PSU Calc"() -> (w1606:T1)
            n506 = Unbundle By Name(w1606) -> ("Low speed (km/s)"=w1605:dbl, "High speed (km/s)"=w1604:dbl, "Window (Delta-T)"=w1599:dbl, "Lower Cutoff"=w1598:dbl, "Multiplier"=w1597:u16, "Low Charge (fC)"=w1602:dbl, "High Charge (fC)"=w1601:dbl, "Low Radius (µm)"=w1574:dbl, "High Radius (µm)"=w1573:dbl, "Exp. Voltage (MV)"=w1565:dbl)  [unwired: 2 out]
            n507 = Multiply(x=w1565, y=1000000.0) -> (x*y=w1564:dbl)
            n508 = Build Array(w1605, w1604) -> (w1603:dbl[])
            n509 = Build Array(w1602, w1601) -> (w1600:dbl[])
            n510 = Build Array(w1574, w1573) -> (w1570:dbl[])
            n511 = Divide(x=w1570, y=1000000.0 ("x")) -> (x/y=w1568:dbl[])
            n512 = Power Of X(1:w1568, 2:3.0 ("x")) -> (0:w1571:dbl[])
            n513 = Divide(x=w1571, y=3.0 ("x")) -> (x/y=w1580:dbl[])
            n514 = Multiply(x=w1580, y=4.0 ("x")) -> (x*y=w1578:dbl[])
            n515 = Multiply(x=w1578, y=3.141592653589793) -> (x*y=w1576:dbl[])
            n516 = Multiply(x=w1576, y=w1575) -> (x*y=w1572:dbl[])
            n517 = case shown="\"Velocity\"" w1582 {
              tunnel: w1603 -> [w1617 _ w1671]
              tunnel: w1564 -> [w1611 w1632 w1661]
              tunnel: w1600 -> [_ w1635 w1663]
              tunnel: w1572 -> [w1619 w1630 w1660]
              tunnel: [w1617 w1626 w1670] -> w1592
              tunnel: [w1609 w1635 w1662] -> w1591
              tunnel: [w1619 w1630 w1659] -> w1590
              tunnel: w1599 -> [w1623 _ w1669]
              tunnel: w1598 -> [w1622 _ w1667]
              tunnel: w1597 -> [w1621 _ w1665]
              tunnel: [w1623 w1638 w1668] -> w1596
              tunnel: [w1622 w1637 w1666] -> w1595
              tunnel: [w1621 w1636 w1664] -> w1594
              tunnel: w1562 -> [_ _ w1658]
              frame "Velocity" {
                n518 = Multiply(x=w1617, y=1000.0 ("Lower Cutoff")) -> (x*y=w1614:dbl[])
                n519 = Divide(x=w1619, y=2.0 ("Lower Cutoff")) -> (x/y=w1615:dbl[])
                n520 = Square(x=w1614) -> (x^2=w1616:dbl[])
                n521 = Multiply(x=w1616, y=w1615) -> (x*y=w1612:dbl[])
                n522 = Divide(x=w1612, y=w1611) -> (x/y=w1610:dbl[])
                n523 = Multiply(x=1000000000000000.0 ("Lower Cutoff"), y=w1610) -> (x*y=w1609:dbl[])
                n524 = local write "Variable 2"(enum32{"Velocity", "Charge", "Mass"}."Mass" ("Variable 2")) -> ()
              }
              frame "Charge" {
                w1645 = 99.989
                w1643 = 1000000.0 ("y")
                n525 = Multiply(x=w1635, y=1e-15 ("x")) -> (x*y=w1633:dbl[])
                n526 = Multiply(x=w1633, y=w1632) -> (x*y=w1631:dbl[])
                n527 = Reverse 1D Array(array=w1630) -> (reversed array=w1624:dbl[])
                n528 = Divide(x=w1631, y=w1624) -> (x/y=w1629:dbl[])
                n529 = Multiply(x=w1629, y=2.0 ("x")) -> (x*y=w1627:dbl[])
                n530 = Square Root(x=w1627) -> (sqrt(x)=w1626:dbl[])
                n531 = Index Array(array=w1626) -> (element #1=w1656:dbl, element #2=w1657:dbl)  [unwired: 2 in]
                n532 = Divide(x=0.6, y=w1656) -> (x/y=w1641:dbl)
                n533 = Divide(x=0.6, y=w1657) -> (x/y=w1642:dbl)
                n534 = Subtract(x=w1641, y=w1642) -> (x-y=w1644:dbl)
                n535 = Multiply(x=w1642, y=w1643) -> (x*y=w1651:dbl)
                n536 = Multiply(x=w1644, y=w1643) -> (x*y=w1650:dbl)
                n537 = Less?(x=w1651, y=w1645) -> (x < y?=w1646:bool)
                n538 = Less?(x=w1650, y=w1645) -> (x < y?=w1647:bool)
                n539 = local write "Variable 2"(enum32{"Velocity", "Charge", "Mass"}."Mass" ("Variable 2")) -> ()
                n540 = And(x=w1646, y=w1647) -> (x .and. y?=w1653:bool)
                n541 = Select(t=u16 0 ("Multiplier"), s=w1653, f=u16 1 ("Multiplier")) -> (s? t:f=w1636:u16)
                n542 = Select(t=10.0, s=w1653, f=1.0) -> (s? t:f=w1652:dbl)
                n543 = Multiply(x=w1650, y=w1652) -> (x*y=w1638:dbl)
                n544 = Multiply(x=w1651, y=w1652) -> (x*y=w1637:dbl)
              }
              frame "Mass" {
                n545 = case shown="\"Mass\"" w1658 {
                  tunnel: w1671 -> [w1674 _ w1727]
                  tunnel: [w1674 w1688 w1727] -> w1670
                  tunnel: w1669 -> [w1678 _ w1726]
                  tunnel: [w1678 w1702 w1726] -> w1668
                  tunnel: w1667 -> [w1677 _ w1725]
                  tunnel: [w1677 w1701 w1725] -> w1666
                  tunnel: w1665 -> [w1676 _ w1724]
                  tunnel: [w1676 w1700 w1724] -> w1664
                  tunnel: w1663 -> [_ w1691 w1723]
                  tunnel: [w1679 w1691 w1723] -> w1662
                  tunnel: [w1672 w1689 w1722] -> w1659
                  tunnel: w1660 -> [w1672 w1689 w1722]
                  tunnel: w1661 -> [w1680 w1690 _]
                  frame "Velocity" {
                    n546 = Multiply(x=w1674, y=1000.0 ("x")) -> (x*y=w1675:dbl[])
                    n547 = Square(x=w1675) -> (x^2=w1684:dbl[])
                    n548 = Divide(x=w1672, y=2.0 ("x")) -> (x/y=w1685:dbl[])
                    n549 = Multiply(x=w1684, y=w1685) -> (x*y=w1683:dbl[])
                    n550 = Divide(x=w1683, y=w1680) -> (x/y=w1682:dbl[])
                    n551 = Multiply(x=1000000000000000.0, y=w1682) -> (x*y=w1679:dbl[])
                  }
                  frame "Charge" {
                    w1715 = 99.989
                    w1717 = 1000000.0 ("y")
                    n552 = Multiply(x=w1691, y=1e-15 ("x")) -> (x*y=w1698:dbl[])
                    n553 = Multiply(x=w1698, y=w1690) -> (x*y=w1697:dbl[])
                    n554 = Reverse 1D Array(array=w1689) -> (reversed array=w1687:dbl[])
                    n555 = Divide(x=w1697, y=w1687) -> (x/y=w1696:dbl[])
                    n556 = Multiply(x=w1696, y=2.0 ("x")) -> (x*y=w1694:dbl[])
                    n557 = Square Root(x=w1694) -> (sqrt(x)=w1692:dbl[])
                    n558 = Index Array(array=w1692) -> (element #1=w1704:dbl, element #2=w1703:dbl)  [unwired: 2 in]
                    n559 = Divide(x=0.6, y=w1704) -> (x/y=w1719:dbl)
                    n560 = Divide(x=0.6, y=w1703) -> (x/y=w1718:dbl)
                    n561 = Subtract(x=w1719, y=w1718) -> (x-y=w1716:dbl)
                    n562 = Multiply(x=w1718, y=w1717) -> (x*y=w1709:dbl)
                    n563 = Multiply(x=w1716, y=w1717) -> (x*y=w1710:dbl)
                    n564 = Less?(x=w1709, y=w1715) -> (x < y?=w1714:bool)
                    n565 = Less?(x=w1710, y=w1715) -> (x < y?=w1713:bool)
                    n566 = Divide(x=w1692, y=1000.0 ("x")) -> (x/y=w1688:dbl[])
                    n567 = And(x=w1714, y=w1713) -> (x .and. y?=w1707:bool)
                    n568 = Select(t=u16 0 ("Multiplier"), s=w1707, f=u16 1 ("Multiplier")) -> (s? t:f=w1700:u16)
                    n569 = Select(t=10.0, s=w1707, f=1.0) -> (s? t:f=w1708:dbl)
                    n570 = Multiply(x=w1710, y=w1708) -> (x*y=w1702:dbl)
                    n571 = Multiply(x=w1709, y=w1708) -> (x*y=w1701:dbl)
                  }
                  frame "Mass" {
                  }
                }
              }
            }
            n572 = Index Array(array=w1592) -> (element #1=w1593:dbl, element #2=w1587:dbl)  [unwired: 2 in]
            n573 = Index Array(array=w1591) -> (element #1=w1589:dbl, element #2=w1588:dbl)  [unwired: 2 in]
            n574 = Index Array(array=w1570) -> (element #1=w1584:dbl, element #2=w1583:dbl)  [unwired: 2 in]
            n575 = Index Array(array=w1590) -> (element #1=w1586:dbl, element #2=w1585:dbl)  [unwired: 2 in]
            n576 = Bundle By Name(cluster=w1606, "Low speed (km/s)"=w1593, "High speed (km/s)"=w1587, "Window (Delta-T)"=w1596, "Lower Cutoff"=w1595, "Multiplier"=w1594, "Low Charge (fC)"=w1589, "High Charge (fC)"=w1588, "Low Mass (kg)"=w1586, "High Mass (kg)"=w1585, "Low Radius (µm)"=w1584, "High Radius (µm)"=w1583, "Exp. Voltage (MV)"=w1565) -> (w1607:T1)
            n577 = local write "PSU Calc"(w1607) -> ()
          }
          event "Accept All Particles": Value Change {
            w1734 = 10.0 ("x")
            w1740 = 0.01 ("x")
            w1741 = 200.0 ("x")
            w1746 = 0.1 ("Low speed (km/s)")
            n578 = event-data() -> ()  [unwired: 1 in, 6 out]
            n579 = property on="PSU Calc" class="Clust (strict)"(error in=w1750) -> (error out=w1749:errorcluster, "Value"=w1748:T1)  [unwired: 1 in, 1 out]
            n580 = Unbundle By Name(w1748) -> ("Low speed (km/s)"=w1745:dbl, "High speed (km/s)"=w1742:dbl, "Low Radius (µm)"=w1738:dbl, "High Radius (µm)"=w1732:dbl)
            n581 = Less?(x=w1746, y=w1745) -> (x < y?=w1747:bool)
            n582 = Select(t=w1746, s=w1747, f=w1745) -> (s? t:f=w1743:dbl)
            n583 = property on="Low speed (km/s)" class="DigNum (strict)"(error in=w1749, "Value"=w1743) -> (error out=w1737:errorcluster)  [unwired: 1 in, 1 out]
            n584 = Greater?(x=w1741, y=w1742) -> (0:w1744:bool)
            n585 = Select(t=w1741, s=w1744, f=w1742) -> (s? t:f=w1731:dbl)
            n586 = property on="High speed (km/s)" class="DigNum (strict)"(error in=w1737, "Val(Sgnl)"=w1731) -> (error out=w1736:errorcluster)  [unwired: 1 in, 1 out]
            n587 = Less?(x=w1740, y=w1738) -> (x < y?=w1739:bool)
            n588 = Select(t=w1740, s=w1739, f=w1738) -> (s? t:f=w1730:dbl)
            n589 = property on="Low Radius (µm)" class="DigNum (strict)"(error in=w1736, "Value"=w1730) -> (error out=w1735:errorcluster)  [unwired: 1 in, 1 out]
            n590 = Greater?(x=w1734, y=w1732) -> (0:w1733:bool)
            n591 = Select(t=w1734, s=w1733, f=w1732) -> (s? t:f=w1729:dbl)
            n592 = property on="High Radius (µm)" class="DigNum (strict)"(error in=w1735, "Val(Sgnl)"=w1729) -> (error out=w1728:errorcluster)  [unwired: 1 in, 1 out]
          }
        }
        n593 = Or(x="PSU update", y="OK1") -> (x .or. y?=w567:bool)
        n594 = Or(x="Cancel", y=w567) -> (x .or. y?=w563:bool)
        n595 = Not(x=w565) -> (.not. x?=w564:bool)
        n596 = Compound Arithmetic op=OR(w564, w562, w563) -> (w561:bool)
        n597 = flat-sequence {
          tunnel: [w571] -> w557
          tunnel: w556 -> [w571]
          tunnel: [w570] -> w555
          frame #0 {
            n598 = local read "PSU Calc"() -> (w570:T1)
          }
        }
        n599 = Wait Until Next ms Multiple(millisecond multiple=u32 50) -> ()  [unwired: 1 out]
      }
      "OK" <- w89
      "Cancel 2" <- w81
      n600 = case shown="False" w81 {
        tunnel: w80 -> [w142 w147]
        tunnel: [w131 w147] -> w16
        tunnel: w79 -> [w146 _]
        frame False {
          n601 = Get Date/Time In Seconds() -> (seconds since 1Jan1904=w140:timestamp)
          n602 = global write "PSU updated.vi" "PSU updated"(TRUE ("PSU updated")) -> ()
          n603 = Unbundle By Name(w146) -> ("Low speed (km/s)"=w144:dbl, "High speed (km/s)"=w143:dbl, "Low Charge (fC)"=w128:dbl, "High Charge (fC)"=w129:dbl, "High Mass (kg)"=w127:dbl, "Low Mass (kg)"=w126:dbl)
          n604 = local read "Variable 1"() -> (w125:enum32{"Velocity", "Charge", "Mass"})
          n605 = local read "Variable 2"() -> (w124:enum32{"Velocity", "Charge", "Mass"})
          n606 = call "timestamp_conversion.vi"("error in (no error)"=w142, "Time Stamp"=w140) -> ("error out"=w139:errorcluster, "Integer Time"=w141:i64)  [unwired: 7 in]
          n607 = Bundle By Name(cluster=T5 {"Integer Timestamp"=0.0, "Max Velocity"=0.0, "Min Velocity"=0.0, "Max Charge"=0.0, "Min Charge"=0.0, "Max Mass"=0.0, "Min Mass"=0.0, "Variable 1"=enum."Mass", "Variable 2"=enum."Mass"} ("PSU settings"), "Integer Timestamp"=w141, "Max Velocity"=w143, "Min Velocity"=w144, "Max Charge"=w129, "Min Charge"=w128, "Max Mass"=w127, "Min Mass"=w126, "Variable 1"=w125, "Variable 2"=w124) -> (w136:T5)
          n608 = call "connect in.vi"("error in (no error)"=w139) -> ("error out"=w134:errorcluster, "Database Connection"=w137:T6)  [unwired: 6 in, 1 out]
          n609 = call <vilib>:"DB Tools Insert Data.vi"("data"=w136, "error in (no error)"=w134, "columns"=string[] [], "table"="psu", "connection reference"=w137) -> ("error out"=w133:errorcluster, "connection reference out"=w135:T6)  [unwired: 5 in]
          n610 = call "connect out.vi"("error in (no error)"=w134, "connection reference"=w135) -> ("error out"=w132:errorcluster)  [unwired: 9 in]
          n611 = Merge Errors(w133, w132) -> (w131:errorcluster)
        }
        frame True {
        }
      }
      n612 = property class="VI"(error in=w16) -> (error out=w15:errorcluster, "FP.State"=w20:T3)  [unwired: 1 in, 1 out]
      n613 = Not Equal?(x=w20, y=T3."Closed") -> (x != y?=w18:bool)
      n614 = And(x="sub vi?", y=w18) -> (x .and. y?=w21:bool)
      n615 = case shown="True" w21 {
        tunnel: w15 -> [w111 w114]
        tunnel: [w111 w113] -> w23
        tunnel: [FALSE ("sub vi?") FALSE ("sub vi?")] -> w17
        frame False {
        }
        frame True {
          n616 = invoke class="VI" method="FP.Close"(error in=w114) -> (error out=w113:errorcluster)  [unwired: 2 in, 2 out]
        }
      }
      n617 = local write "sub vi?"(w17) -> ()
    }
    frame Error {
    }
  }
  "error out" <- w10
